vi "main.vi"(0 "Test Pins":T6, 1 "Caller Information":T7, 5 "Test Inputs":T10={"Load Current 1 in A"=0.0, "Load Current 2 in A"=0.0, "Duration of the pulse in Second"=0.5, "Nominal Output Voltage in V"=0.0, "Ref Voltage level for Settling Time Calc"=0.1, "% of Vnom for Settling Time Calc"=10.0, "Settling Time Calc Option"=enum."Voltage Level ", "Advance Setting"={"Prepare"={"Power Test Board.Voltage Level (V)"=6.0, "Power Test Board.Current Limit (A)"=0.1, "Sense Resistance (Ohm)"=1.0, "Fgen.Sample Rate (Sample/s)"=20000000.0}, "Stimulus And Measure"={"Fgen.Offset (V)"=0.0}}, "Save Transient Graph?"=TRUE, "Input Voltage in V"=0.0, "Save Scope Raw Data?"=FALSE, "Delay - t1 in s"=0.25, "Delay - t2 in s"=0.25, "Auto Scale Y-Axis?"=TRUE, "Shunt Resistance (Ohm)"=1.0, "Slew Rate (A/us)"=0.001, "Measure Rising Edge Slew Rate?"=TRUE, "Measure Falling Edge Slew Rate?"=TRUE} {"Advance Setting"."Stimulus And Measure"."Fgen.Offset (V)" min=1.0 format="%#_6p"; "Advance Setting"."Prepare"."Power Test Board.Current Limit (A)" min=1.0 format="%#_6p"; "Advance Setting"."Prepare"."Power Test Board.Voltage Level (V)" min=1.0 format="%#_6p"; "Advance Setting"."Prepare"."Fgen.Sample Rate (Sample/s)" min=1.0 format="%#_6p"; "Advance Setting"."Prepare"."Sense Resistance (Ohm)" min=1.0 format="%#_6p"}, 11 "error in":errorcluster) -> (4 "Test Results":T15 {"Falling Edge - Measured Slew Rate (A/us)" format="%#.5p"; "Rising Edge - Measured Slew Rate (A/us)" format="%#.5p"; "Second Edge - Settling Time in s" format="%#.5p"; "First Edge - Settling Time in s" format="%#.5p"; "Actual Sample Rate in S/s" format="%#.5g"}, 15 "error out":errorcluster)   [LabVIEW 2020, in "LDO Load Transient_AWG.lvlib"]
doc: "<b>Caller</b> Information is input for framework components. Mode should be set to <b>Automation</b> when running from TestStand. Sequence Context should be set to <b>ThisContext</b> when running from TestStand. The values will be updated everytime the setting is applied using \"Edit\" dialog.\n\n<b>Test Pins</b> is names of pins available in the pinmap file. Provide the right pins for the required functionality.\n\n<b>Test Inputs</b> is input required for the measurement to perform.\n\n<b>error in</b> is meant for the sequencing. <b>error in</b> should be <b>no error</b> always.\n\n<b>Test Results</b> contains all the measured data during the measurement and processed results.\n\n<b>error out</b> contains the error occured during measurement.\n\nCheck measurement documentation for more information (<Program Files>\\Soliton Technologies\\MeasurementSuite\\CodeModules\\LDO\\LDO Load Transient.pdf)"
uses:
  LDO Load Transient_AWG.lvlib
  Typedefs/Test Results.ctl
  Typedefs/Test Inputs.ctl
  Typedefs/Settling Time Calc Option.ctl
  Typedefs/Advance Settings.ctl
  Typedefs/Adv Settings Setup Instr.ctl
  Typedefs/Adv Settings Stimulus and Measure.ctl
  <userlib>/_Soliton/Measurement Suite/Reusables/Plugin Common/Typedefs/Caller Events.ctl
  <userlib>/_Soliton/Measurement Suite/Reusables/Plugin Common/Typedefs/Caller Information.ctl
  <userlib>/_Soliton/Measurement Suite/Reusables/Plugin Common/Typedefs/Caller Mode.ctl
  Typedefs/Test Pins.ctl
  Typedefs/Pin Dropdown.ctl
  <userlib>/_Soliton/Measurement Suite/Reusables/Plugin Common/Typedefs/Termination Monitor Info.ctl
  Reusables/UI/Progress Monitor/Progress Monitor Option.ctl
  <vilib>/Utility/miscctls.llb/LVMajorAndMinorColorsTypeDef.ctl
  <instrlib>/niDCPower/nidcpower.llb/niDCPower Source Mode.ctl
  <instrlib>/niDCPower/nidcpower.llb/niDCPower Output Function.ctl
  <instrlib>/niDCPower/nidcpower.llb/niDCPower Wait For Event - Event.ctl
  <instrlib>/niFgen/niFgen.llb/niFgen Trigger Mode.ctl
  <instrlib>/niFgen/niFgen.llb/niFgen Output Mode.ctl
  Typedefs/Transient Configuration.ctl
  <instrlib>/niScope/Controls/niScope scalar measurement.ctl
  <vilib>/Utility/error.llb/DialogType.ctl
  c0d3c9e0-367a-4754-9b2e-773ed4fafa93.vi
  d648f1df-a8d9-4085-9eb0-24252e83c66e.vi
  98c31a9a-65c4-404a-8d29-5fef3c3d30dc.vi
  293d3250-dd4c-4630-9c2a-ad0ba4e4c4de.vi
  e89c743e-5273-4ded-a4f4-1d44fefc8133.vi
  44f97677-0516-4608-8e28-d738a12fef77.vi
  01e50ca5-2bbf-454e-9d2d-d5f5dbc62a55.vi
  49732470-67c5-4264-8b59-91d7a6bf13ef.vi
  29f2f23f-c0b0-483c-8177-98a50cbfcdf1.vi
  a7f9c5ee-455a-46a4-a79d-0a7db08c4ebb.vi
  bb3e62c4-a2c2-4505-9438-f842dd651d6c.vi
  ce2ee1e5-697c-4608-b941-8c9b0f21ffd9.vi
  217e438d-a1ad-49ce-9dcd-d015b5ab8206.vi
  3210b59a-1980-40a2-8b26-190a43568d65.vi
  eadbd7cd-77f9-412a-9e87-0f7f53d679d4.vi
  <userlib>/_Soliton/Measurement Suite/Reusables/InstrumentSessionAPIs/SessionManagerApiPath.vi
  <vilib>/Utility/sysdir.llb/Get System Directory.vi
  <vilib>/Utility/LVLibp/Get Exported File Path.vi
  <userlib>/_Soliton/Measurement Suite/Reusables/Errors/Error 6001.vi
  <instrlib>/niScope/Measurements/niScope Fetch Measurement.vi
  <userlib>/_Soliton/Measurement Suite/Reusables/Plugin Common/Plugin Common.lvlib
  <userlib>/_Soliton/Measurement Suite/Reusables/Queue Driver/Plugin Queue Driver.lvlib
panel:
  out "Progress":i32(slide) scale=-1.0..17.0
  in  "Terminate":bool
  in  "Run":bool caption="Measure"
  in  "Exit":bool
  out "Header":string
  in  "Tab Enum":T1(radio)
  out "Tab Control":T2(tab)
  in  "SystemSetup":T4={"Power test Board"={"PinStatus"=0, "PinName"="", "Info"=TRUE}, "Set Input Voltage"={"PinStatus"=0, "PinName"="", "Info"=TRUE}, "Measure Output Voltage"={"PinStatus"=0, "PinName"="", "Info"=TRUE}, "Measure Load Current"={"PinStatus"=0, "PinName"="", "Info"=TRUE}, "Set Arbitrary Waveform"={"PinStatus"=0, "PinName"="", "Info"=TRUE}}
  in  "Shunt Resistance (Ohm)":dbl=1.0 min=1.0 format="%#_6p"
  out "Shunt Resistance Info":u16(ring) caption="Set 1 Ohm if its Current Probe"
  in  "Slew Rate (A/us)":dbl format="%#_6p"
  out "Sequence Timeout":dbl caption="Sequence Timeout (s)" format="%#.5p"
  in  "Delay - t2 (s)":dbl=0.25 format="%#_6p"
  in  "Delay - t1 (s)":dbl=0.25 format="%#_6p"
  in  "Duration of the pulse (s)":dbl=0.5 format="%#_6p"
  in  "Percentage of Vnom (%)":dbl=10.0 caption="Percentage of nominal voltage (%)" format="%#_6f"
  in  "Voltage to settle above Vnom (V)":dbl=0.1 format="%#_6p"
  in  "Load Current 1 - Iload1 (A)":dbl format="%#_6p"
  in  "Settling Time Calculation":enum32{"Item 0", "Item 1"}(radio)
  in  "Input Voltage (V)":dbl format="%#_6p"
  in  "Load Current 2 - Iload2 (A)":dbl format="%#_6p"
  in  "Nominal Output Voltage (V)":dbl format="%#_6p"
  in  "Advanced Settings":bool
  in  "Measure Falling Edge Slew Rate?":bool=TRUE
  in  "Measure Rising Edge Slew Rate?":bool=TRUE
  out "Falling Edge - Measured Slew Rate (A/us)":dbl format="%#.5p"
  out "Rising Edge - Measured Slew Rate (A/us)":dbl format="%#.5p"
  out "Second Edge - Settling Time (s)":dbl format="%#.5p"
  in  "Auto Scale Y-Axis?":bool=TRUE
  in  "Save Scope Raw Data?":bool=TRUE
  out "Load Transient":cluster{"x-axis":dbl[], "wfm":dbl[]}[](graph)
  in  "Take Transient snapshot?":bool=TRUE
  out "Transient Load Current":waveform(dbl)(graph)
  out "Transient Output Voltage":T5(graph)
  out "First Edge - Settling Time (s)":dbl format="%#.5p"
  out "Rising Edge not found?":bool
  out "Falling Edge not found?":bool
  in  "Caller Events":T9
  in  "DataLogPath":path
  in  "ErrorOccured":errorcluster
  # "Supports NIScopeInstrument"
  # "Supports NIScopeInstrument"
  # "Supports NIDCPowerInstrument"
  # "Supports NIFGenInstrument"
  # "Supports NIDCPowerInstrument"
  # "Load Current"
  # "Minimum value for Delay-t1, Duration of the pulse, Delay-t2 should be larger than [ ( Souredelay+Aperture Time ) x Record Length ]"
  # "Settling Time Calculation"
  # "Settling Time is defined as the time taken for the output voltage to recover\nto the LDO nominal output voltage."
  # "Time taken for output voltage to settle to (Choose one below)"
  # "Load Transient"
  # "Output Voltage"
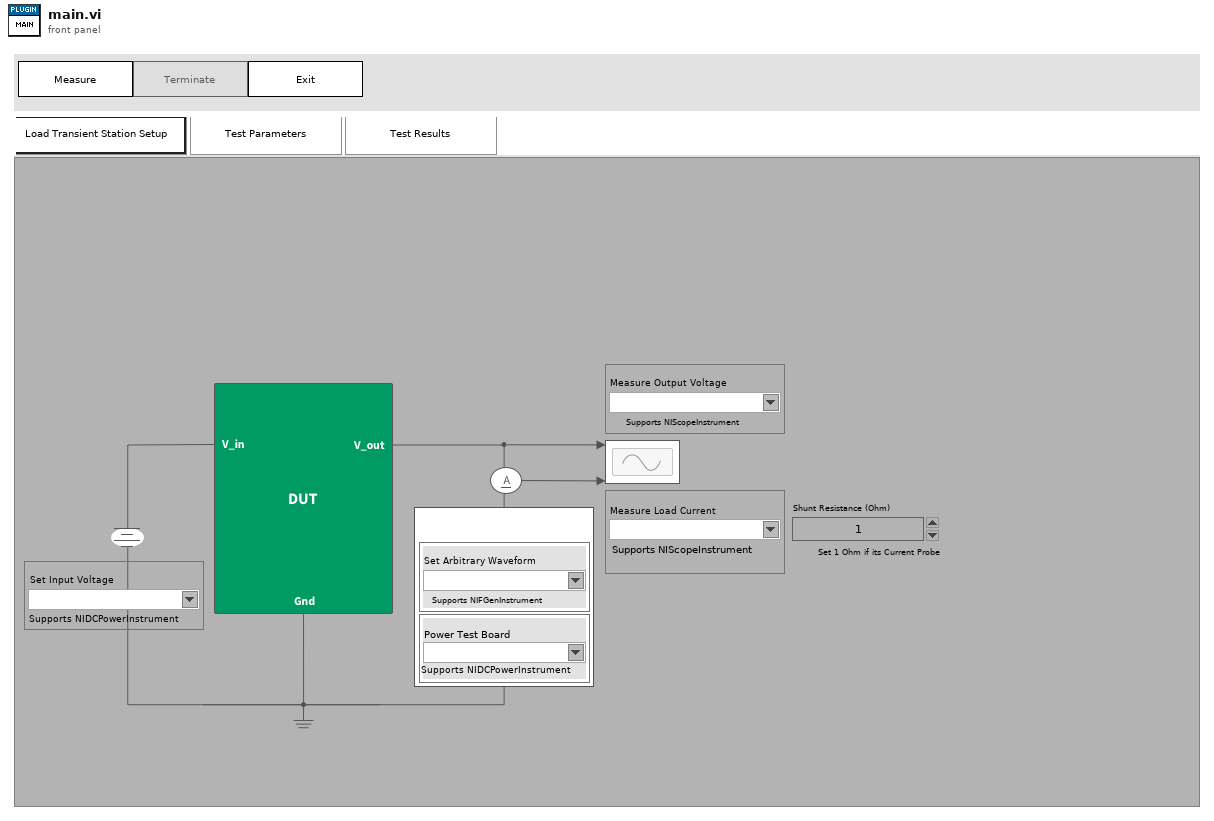
[diagram p1: front panel]
types:
  T1 = enum32{"Station Setup", "Test Parameters", "Test Results"}
  T2 = enum32{"Station Setup", "Test Parameters", "Test Results", "Debug"}
  T3 = typedef "LDO Load Transient_AWG.lvlib/Pin Dropdown.ctl" = cluster{"PinStatus":u16, "PinName":string, "Info":bool}
  T4 = cluster{"Power test Board":T3, "Set Input Voltage":T3, "Measure Output Voltage":T3, "Measure Load Current":T3, "Set Arbitrary Waveform":T3}
  T5 = cluster{"relativeInitialX":dbl, "xIncrement":dbl, "wfm":dbl[]}
  T6 = typedef "LDO Load Transient_AWG.lvlib/Test Pins.ctl" = cluster{"Set Input Voltage":string, "Set Load Current":string, "Set Arbitrary Waveform":string, "Measure Output Voltage":string, "Measure Load Current":string}
  T7 = typedef "Plugin Common.lvlib/Caller Information.ctl" = cluster{"Mode":T8, "Sequence Context":refnum<k7>}
  T8 = typedef "Plugin Common.lvlib/Caller Mode.ctl" = enum16{"Standalone", "Automation", "MeasurementSuite"}
  T9 = typedef "Plugin Common.lvlib/Caller Events.ctl" = cluster{"Caller Event":refnum<user-event>}
  T10 = typedef "LDO Load Transient_AWG.lvlib/Test Inputs.ctl" = cluster{"Load Current 1 in A":dbl, "Load Current 2 in A":dbl, "Duration of the pulse in Second":dbl, "Nominal Output Voltage in V":dbl, "Ref Voltage level for Settling Time Calc":dbl, "% of Vnom for Settling Time Calc":dbl, "Settling Time Calc Option":T11, "Advance Setting":T12, "Save Transient Graph?":bool, "Input Voltage in V":dbl, "Save Scope Raw Data?":bool, "Delay - t1 in s":dbl, "Delay - t2 in s":dbl, "Auto Scale Y-Axis?":bool, "Shunt Resistance (Ohm)":dbl, "Slew Rate (A/us)":dbl, "Measure Rising Edge Slew Rate?":bool, "Measure Falling Edge Slew Rate?":bool}
  T11 = typedef "LDO Load Transient_AWG.lvlib/Settling Time Calc Option.ctl" = enum16{"Voltage Level ", "Percentage of Vnom"}
  T12 = typedef "LDO Load Transient_AWG.lvlib/Advance Settings.ctl" = cluster{"Prepare":T13, "Stimulus And Measure":T14}
  T13 = typedef "LDO Load Transient_AWG.lvlib/Adv Settings Setup Instr.ctl" = cluster{"Power Test Board.Voltage Level (V)":dbl, "Power Test Board.Current Limit (A)":dbl, "Sense Resistance (Ohm)":dbl, "Fgen.Sample Rate (Sample/s)":dbl}
  T14 = typedef "LDO Load Transient_AWG.lvlib/Adv Settings Stimulus and Measure.ctl" = cluster{"Fgen.Offset (V)":dbl}
  T15 = typedef "LDO Load Transient_AWG.lvlib/Test Results.ctl" = cluster{"Measured Output Voltage":cluster{"x-axis":dbl[], "wfm":dbl[]}, "Measured Load Current":cluster{"x-axis":dbl[], "wfm":dbl[]}, "Actual Sample Rate in S/s":dbl, "First Edge - Settling Time in s":dbl, "Second Edge - Settling Time in s":dbl, "Rising Edge - Measured Slew Rate (A/us)":dbl, "Falling Edge - Measured Slew Rate (A/us)":dbl}
  T16 = typedef "Plugin Common.lvlib/Termination Monitor Info.ctl" = cluster{"Caller Information":T7, "Execution":refnum<k7>, "Termination Monitor":refnum<k7>, "Type":string, "Plugin Name":string}
  T17 = cluster{"Termination Monitor Info":T16, "Test Inputs":T10, "Test Results":T15, "Test Results[][]":string[][], "Test Pins":T6, "Logger Folder Path":path, "Valid Logger Path?":bool, "Logger File Path":path, "Min delay for Reference Position":u32, "Output Voltage Coupling":i32, "UI Ctls":refnum<vi>[], "Insufficient memory?":bool, "Scope Channels":string, "Scope Acquired time(s)":dbl, "Rising Edge not found?":bool, "Falling Edge not found?":bool}
  T18 = typedef "Progress Monitor Option.ctl" = enum16{"State Array Init", "Get State Index"}
  T19 = enum8{"Enabled", "Disabled", "Disabled and Grayed Out"}
  T20 = typedef "LDO Load Transient_AWG.lvlib/Transient Configuration.ctl" = cluster{"Delay - t1 (s)":dbl, "Duration of the pulse (s)":dbl, "Delay - t2 (s)":dbl, "Load Current 1 - Iload1 (A)":dbl, "Load Current 2 - Iload2 (A)":dbl, "Slew rate A/us":dbl, "Sense Resistance (Ohm)":dbl}
  T21 = typedef "LVMajorAndMinorColorsTypeDef.ctl" = cluster{"Major Color":u32, "Minor Color":u32}
  T22 = typedef "niDCPower Wait For Event - Event.ctl" = i32
  T23 = typedef "niDCPower Output Function.ctl" = i32
  T24 = typedef "niDCPower Source Mode.ctl" = i32
  T25 = typedef "niFgen Output Mode.ctl" = u32
  T26 = typedef "niFgen Trigger Mode.ctl" = i32
  T27 = typedef "niScope scalar measurement.ctl" = i32
  T28 = typedef "DialogType.ctl" = u16
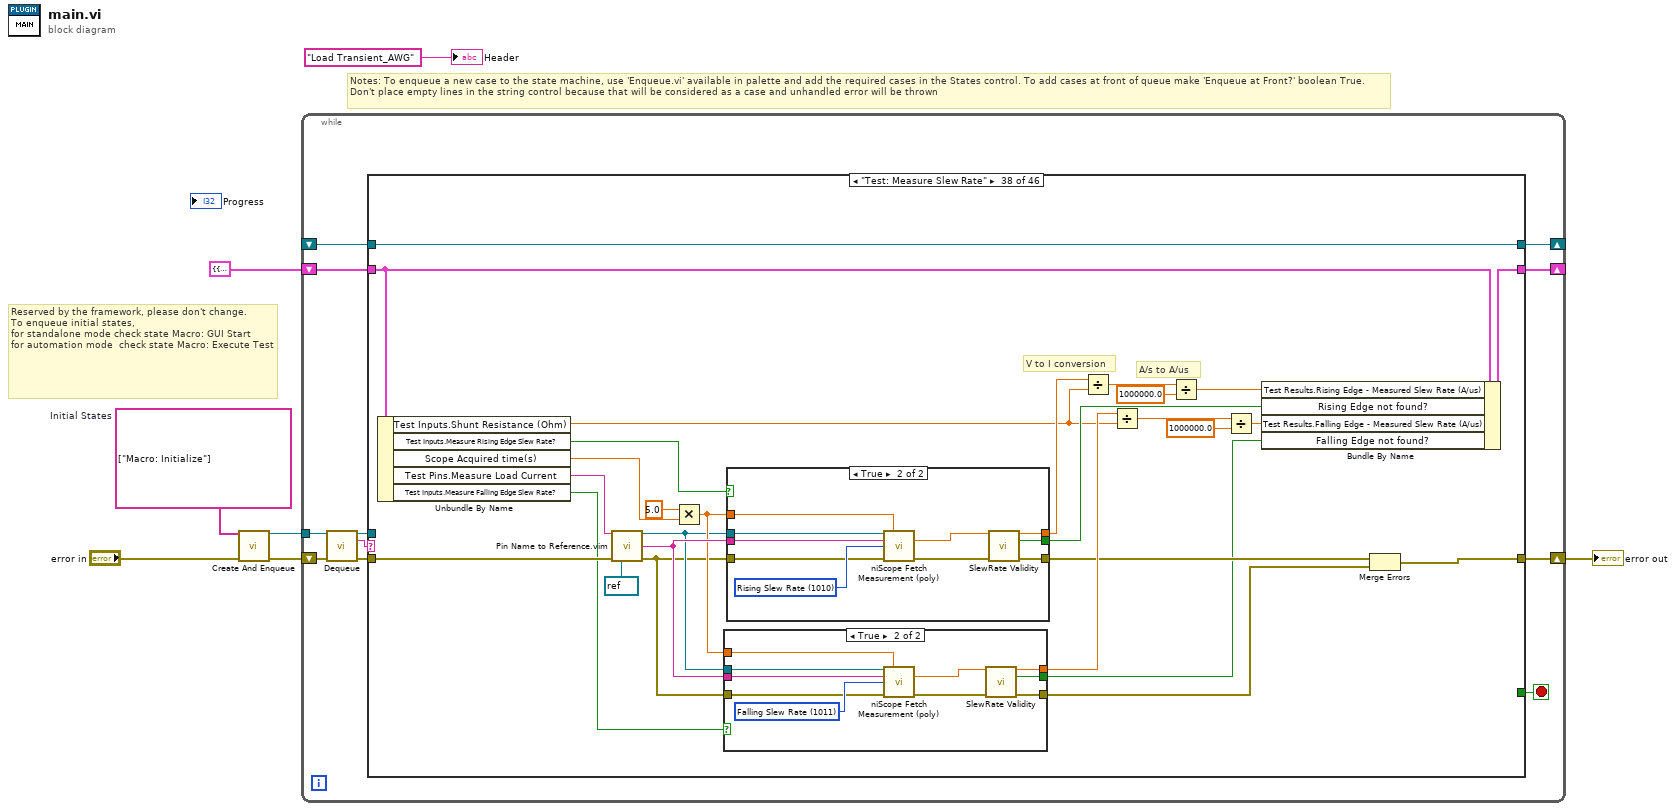
[diagram p0: block diagram]
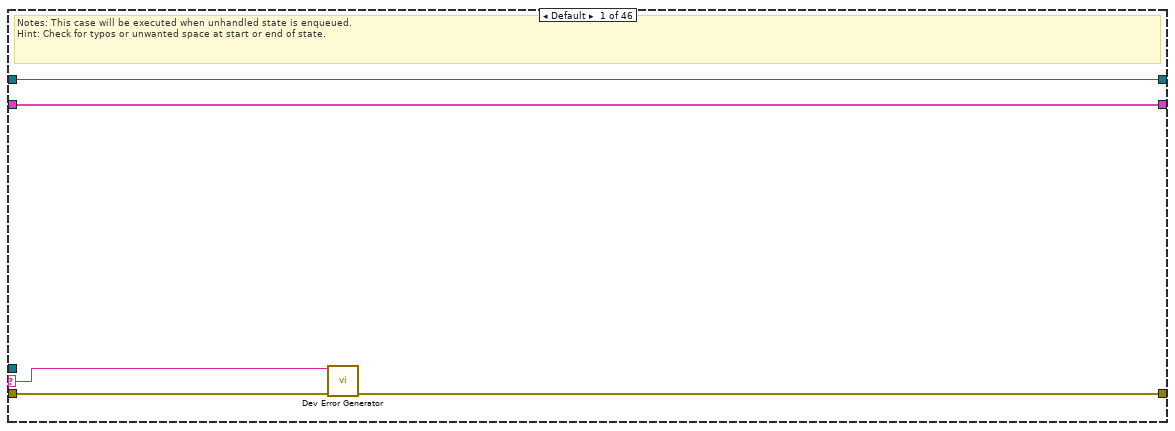
[diagram p2: hidden frame]
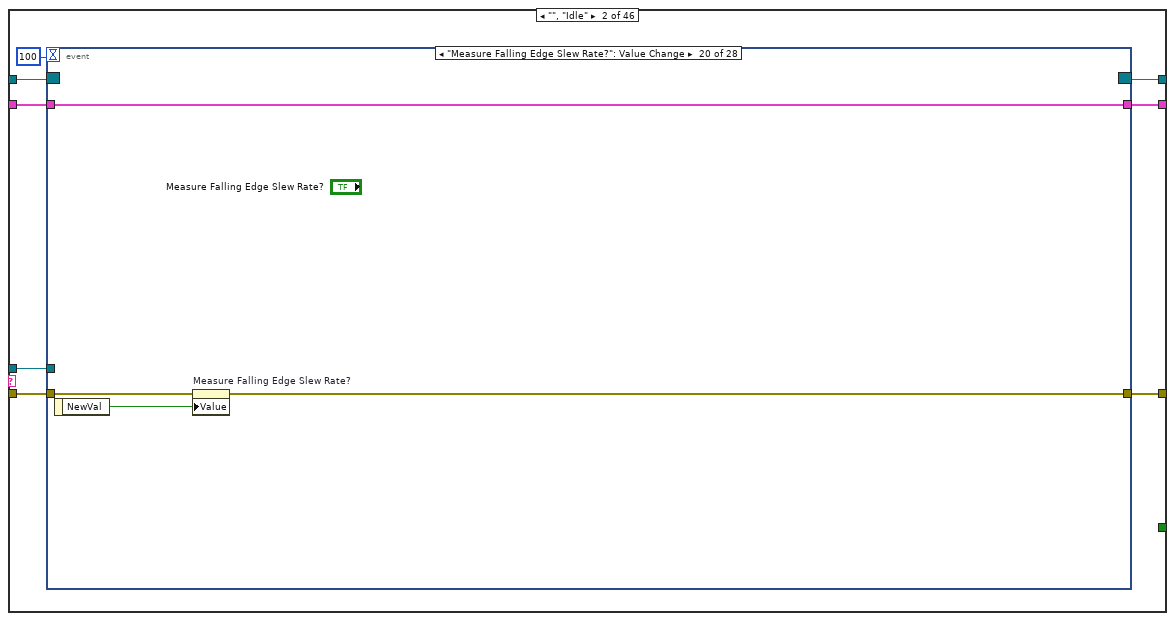
[diagram p3: hidden frame]
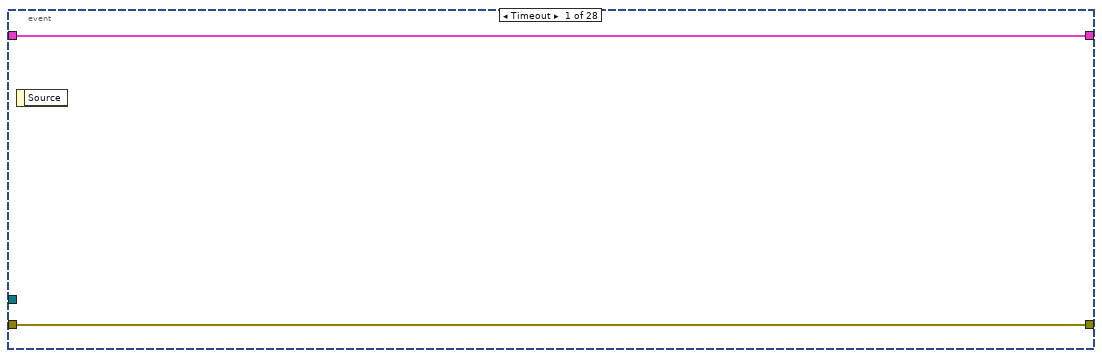
[diagram p4: hidden frame]
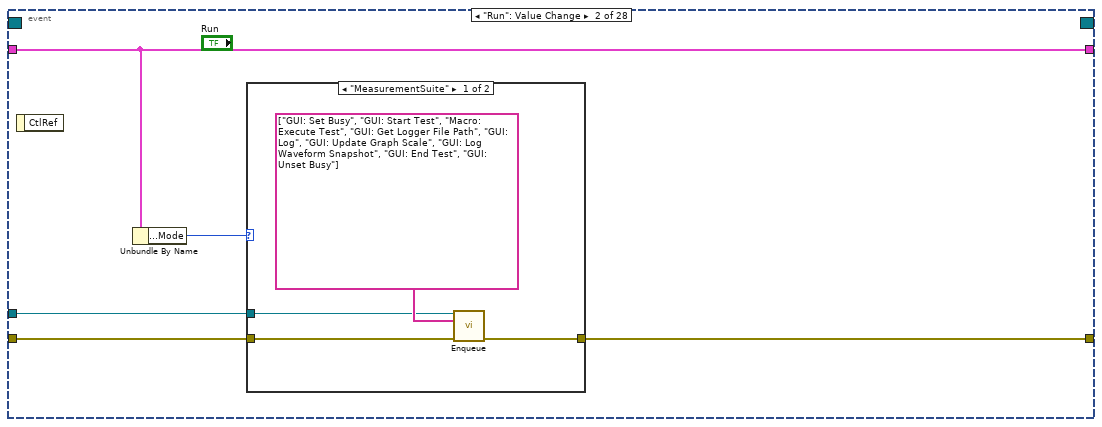
[diagram p5: hidden frame]
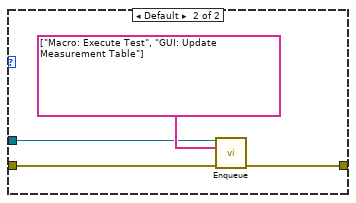
[diagram p6: hidden frame]
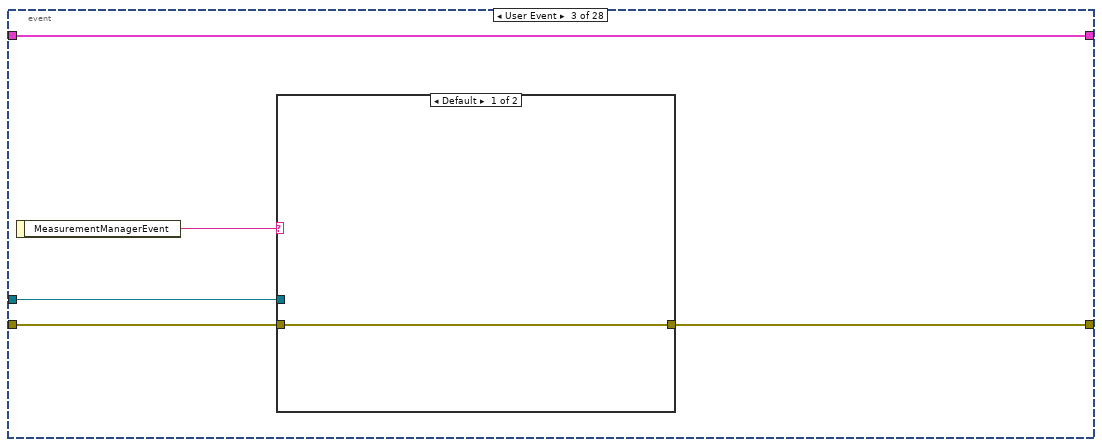
[diagram p7: hidden frame]
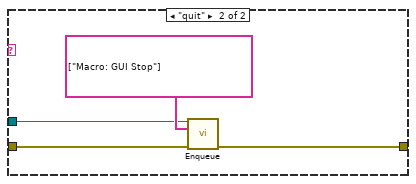
[diagram p8: hidden frame]
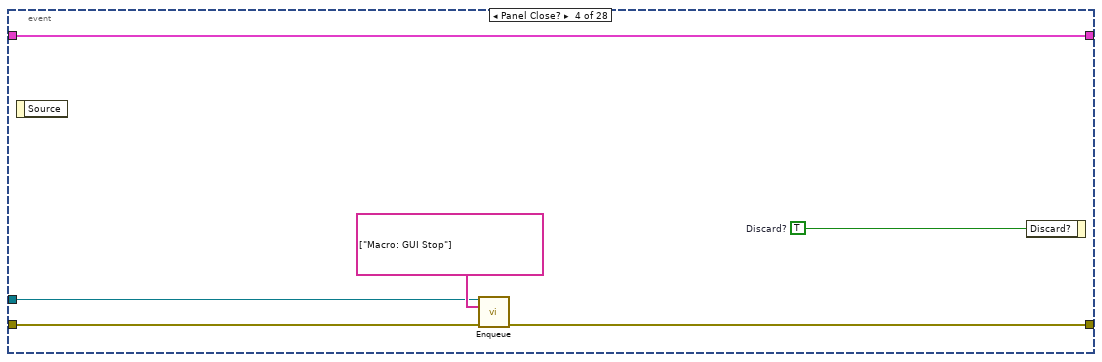
[diagram p9: hidden frame]
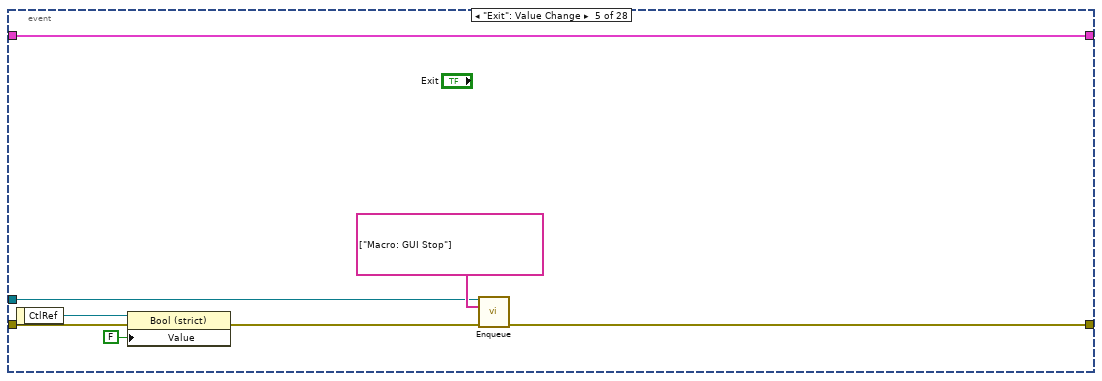
[diagram p10: hidden frame]
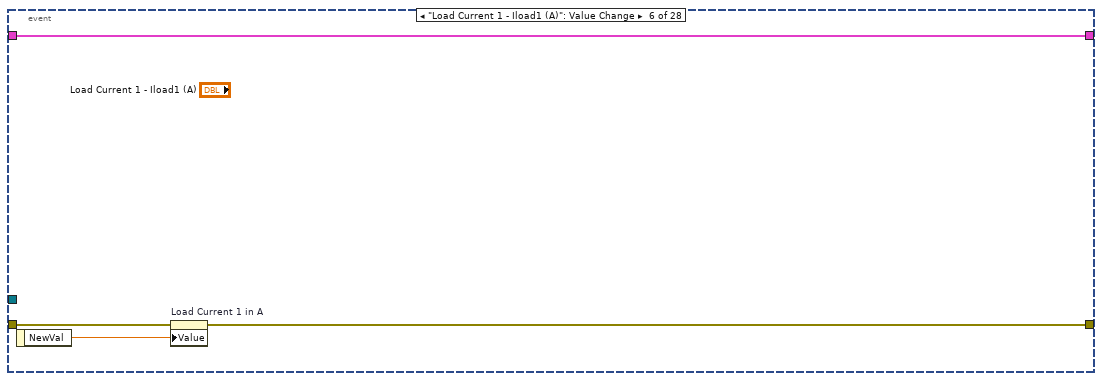
[diagram p11: hidden frame]
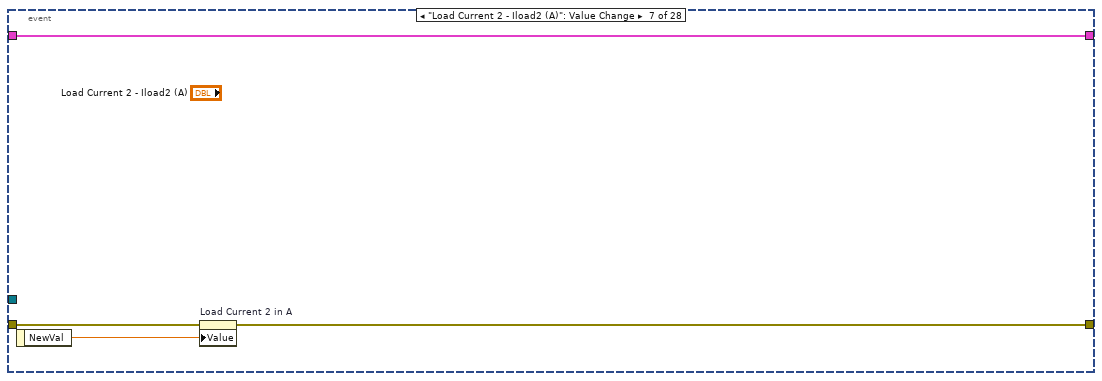
[diagram p12: hidden frame]
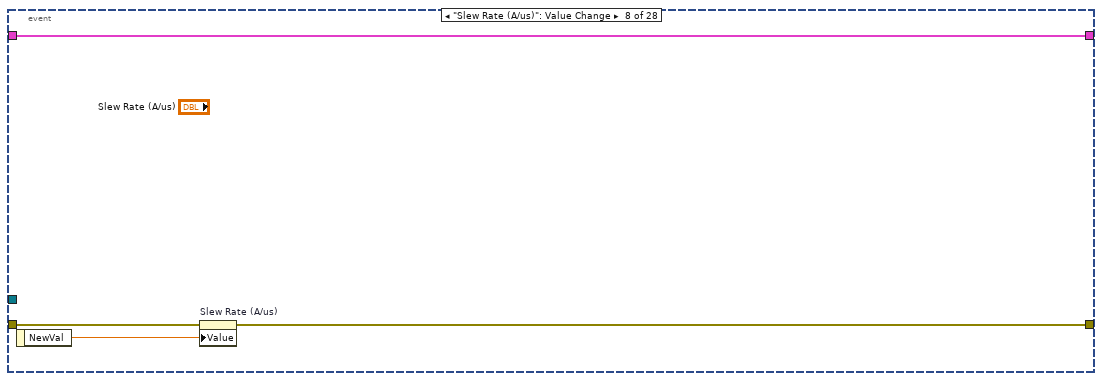
[diagram p13: hidden frame]
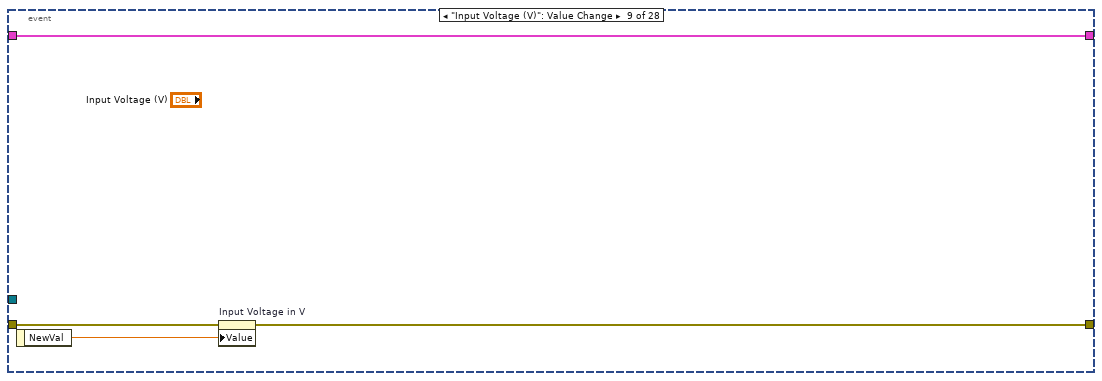
[diagram p14: hidden frame]
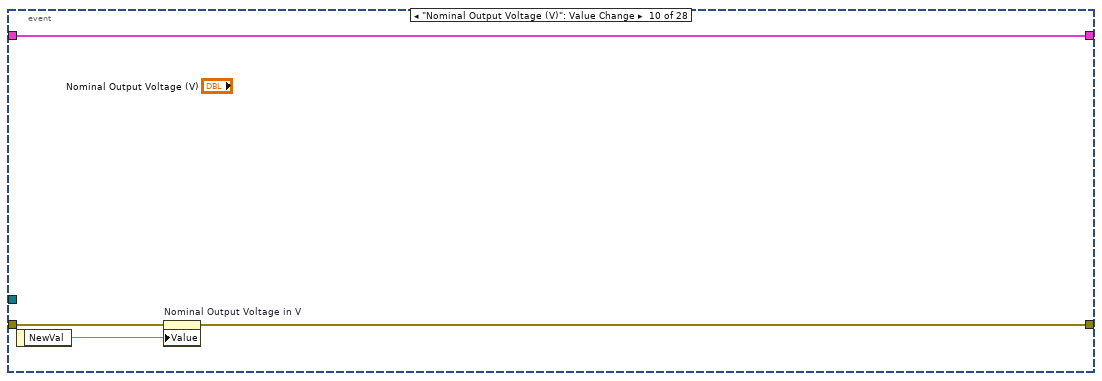
[diagram p15: hidden frame]
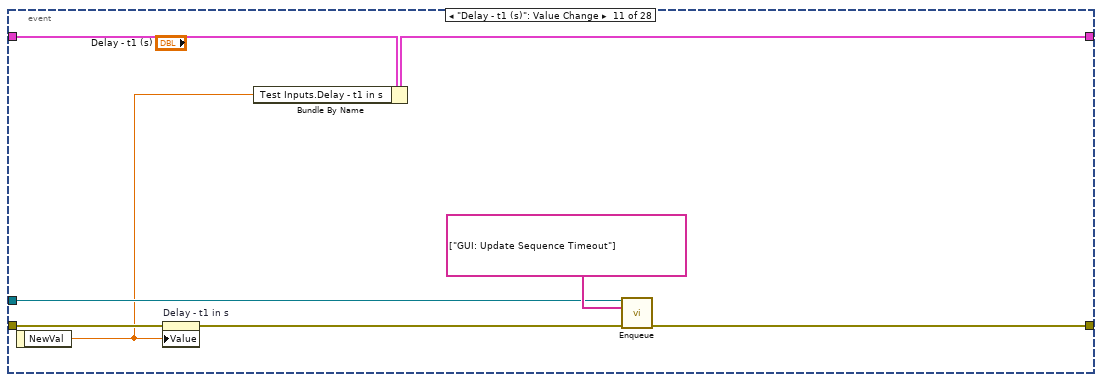
[diagram p16: hidden frame]
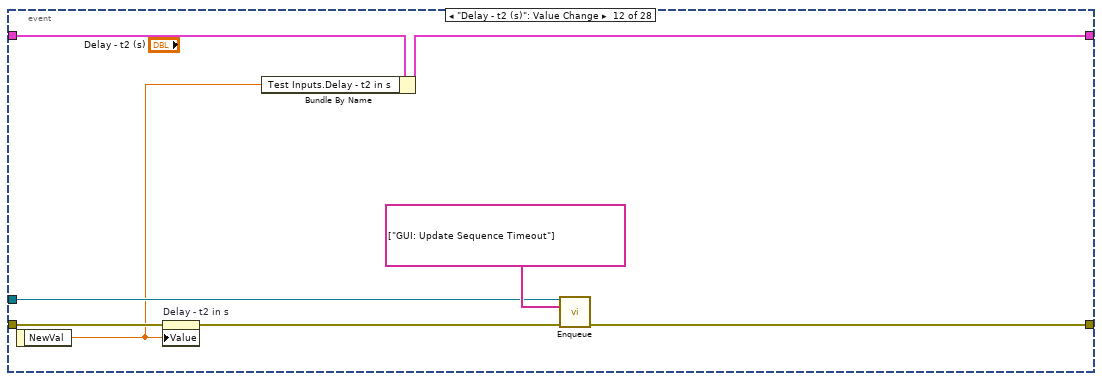
[diagram p17: hidden frame]
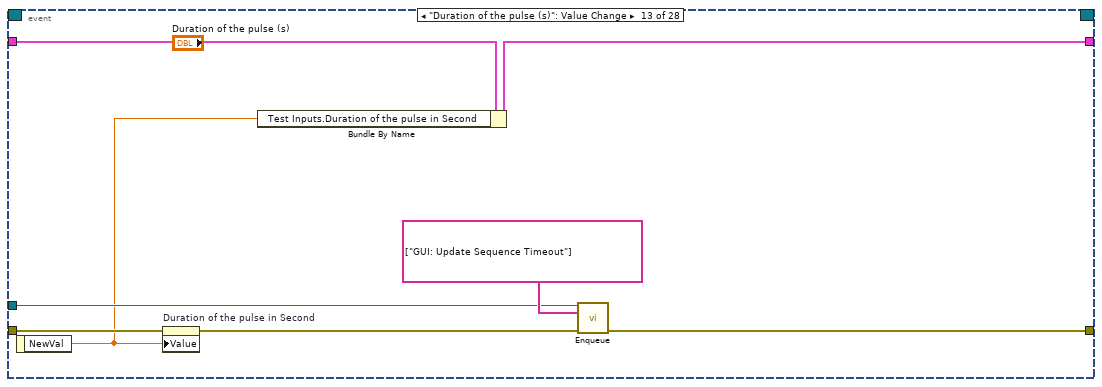
[diagram p18: hidden frame]
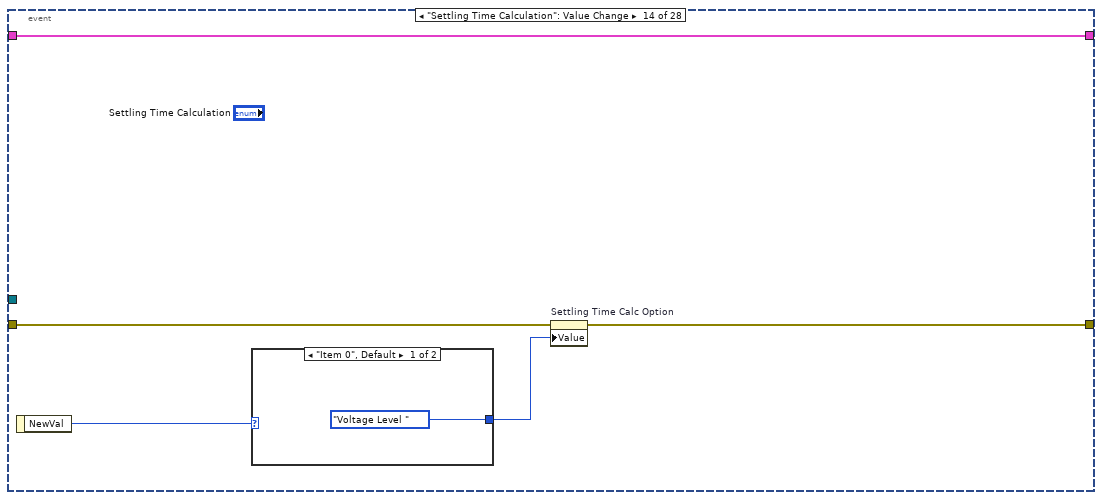
[diagram p19: hidden frame]
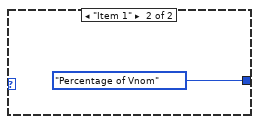
[diagram p20: hidden frame]
diagram:
  w7 = string[] ["Macro: Initialize"]  # Initial States
  # "Notes: To enqueue a new case to the state machine, use 'Enqueue.vi' available in palette and add the required cases in the States control. To add cases at front of queue make 'Enqueue at Front?' boolean True. Don't place empty lines in the string control because that will be considered as a case and unhandled error will be thrown"
  # "Reserved by the framework, please don't change. \nTo enqueue initial states,\nfor standalone mode check state Macro: GUI Start\nfor automation mode  check state Macro: Execute Test"
  n1 = call <userlib>:"Create And Enqueue.vi"("Initial States"=w7, "error in (no error)"="error in") -> ("Queue out"=w5:refnum<queue>, "error out"=w3:errorcluster)  [unwired: 12 in]
  n2 = while {
    shift-right: [w18] -> w4
    shift-left: w3 -> [w16]
    shift-right: [w14] -> _
    shift-left: T17 {"Termination Monitor Info"={"Caller Information"={"Mode"=enum."Standalone", "Sequence Context"=refnum}, "Execution"=refnum, "Termination Monitor"=refnum, "Type"="", "Plugin Name"=""}, "Test Inputs"={"Load Current 1 in A"=0.0, "Load Current 2 in A"=0.0, "Duration of the pulse in Second"=0.0, "Nominal Output Voltage in V"=0.0, "Ref Voltage level for Settling Time Calc"=0.0, "% of Vnom for Settling Time Calc"=0.0, "Settling Time Calc Option"=enum."Voltage Level ", "Advance Setting"={"Prepare"={"Power Test Board.Voltage Level (V)"=0.0, "Power Test Board.Current Limit (A)"=0.0, "Sense Resistance (Ohm)"=1.0, "Fgen.Sample Rate (Sample/s)"=1.0}, "Stimulus And Measure"={"Fgen.Offset (V)"=0.0}}, "Save Transient Graph?"=FALSE, "Input Voltage in V"=0.0, "Save Scope Raw Data?"=FALSE, "Delay - t1 in s"=0.0, "Delay - t2 in s"=0.0, "Auto Scale Y-Axis?"=FALSE, "Shunt Resistance (Ohm)"=0.0, "Slew Rate (A/us)"=0.0, "Measure Rising Edge Slew Rate?"=TRUE, "Measure Falling Edge Slew Rate?"=TRUE}, "Test Results"={"Measured Output Voltage"={"x-axis"=[], "wfm"=[]}, "Measured Load Current"={"x-axis"=[], "wfm"=[]}, "Actual Sample Rate in S/s"=0.0, "First Edge - Settling Time in s"=0.0, "Second Edge - Settling Time in s"=0.0, "Rising Edge - Measured Slew Rate (A/us)"=0.0, "Falling Edge - Measured Slew Rate (A/us)"=0.0}, "Test Results[][]"=[], "Test Pins"={"Set Input Voltage"="", "Set Load Current"="", "Set Arbitrary Waveform"="", "Measure Output Voltage"="", "Measure Load Current"=""}, "Logger Folder Path"=path "", "Valid Logger Path?"=FALSE, "Logger File Path"=path "", "Min delay for Reference Position"=0, "Output Voltage Coupling"=0, "UI Ctls"=[], "Insufficient memory?"=FALSE, "Scope Channels"="", "Scope Acquired time(s)"=0.0, "Rising Edge not found?"=FALSE, "Falling Edge not found?"=FALSE} -> [w13]
    tunnel: w5 -> [w12]
    shift-right: [w9] -> _
    shift-left: _ -> [w10]
    stop <- w17 stop-if-true
    n3 = call <userlib>:"Dequeue.vi"("Queue in"=w12, "error in (no error)"=w16) -> ("Queue out"=w11:refnum<queue>, "Dequeued State"=w8:string, "error out"=w15:errorcluster)  [unwired: 11 in]
    n4 = case shown="\"Test: Measure Slew Rate\"" w8 {
      selector: w8 -> [w21 _ _ _ _ _ _ _ _ _ _ _ w351 w367 _ _ _ _ _ _ _ _ _ _ _ w529 w549 w582 w613 _ _ w673 w680 w728 w767 w790 w806 _ w889 w906 w924 w940 w949 _ _ _]
      tunnel: w15 -> [w20 w28 w255 w264 w279 w285 w292 w297 w332 w343 w347 w350 w352 w369 w384 w396 w425 w438 w459 w491 w500 w511 w516 w523 w528 w530 w550 w583 w614 w634 w657 w674 w681 w729 w768 w791 w807 w846 w890 w907 w925 w941 w950 w957 w964 w982]
      tunnel: [w22 w29 w255 w267 w270 w286 w293 w297 w298 w341 w345 w350 w356 w372 w385 w395 w426 w436 w460 w492 w499 w511 w517 w524 w528 w536 w548 w562 w617 w620 w658 w672 w688 w714 w764 w792 w808 w830 w883 w910 w919 w942 w951 w957 w962 w976] -> w18
      tunnel: [_ _ _ _ _ _ _ _ _ _ _ _ _ _ _ _ _ _ _ _ _ _ _ _ _ _ _ _ _ _ _ _ _ _ _ _ _ _ _ _ _ _ _ _ w959 TRUE] -> w17
      tunnel: [w23 w31 w254 w257 w280 w287 w294 w296 w323 w342 w346 w349 w355 w371 w391 w394 w427 w452 w458 w498 w508 w510 w515 w522 w527 w535 w553 w585 w612 w637 w660 w677 w685 w731 w771 w795 w811 w839 w895 w912 w929 w947 w954 w956 w961 w983] -> w14
      tunnel: w13 -> [w23 w30 w254 w268 w280 w287 w294 w296 w337 w342 w346 w349 w355 w371 w391 w393 w427 w452 w458 w498 w508 w510 w514 w521 w527 w545 w553 w585 w611 w637 w659 w677 w684 w731 w770 w794 w810 w838 w895 w912 w929 w947 w954 w956 w961 w983]
      tunnel: w11 -> [_ w24 _ w266 w278 w283 w290 _ _ _ _ _ _ _ _ _ _ _ _ _ _ _ _ _ _ _ _ _ _ _ _ _ _ _ _ _ _ _ _ _ _ _ _ _ w958 w981]
      tunnel: w10 -> [w19 w26 w253 w265 w277 w282 w289 w295 w336 _ w344 w348 w362 w378 w392 w401 w428 w453 w465 w497 w507 w509 w518 w525 w526 w543 w554 w586 w619 w638 w661 w678 w689 w732 w772 w801 w820 w848 w896 w917 w932 w948 w953 w955 w963 w980]
      tunnel: [w19 w25 w253 w265 w277 w282 w289 w295 w336 w340 w344 w348 w362 w378 w392 w401 w428 w453 w465 w497 w507 w509 w518 w525 w526 w543 w554 w586 w619 w638 w661 w678 w689 w732 w772 w801 w820 w848 w896 w917 w932 w948 w953 w955 w963 w980] -> w9
      frame Default {
        # "Notes: This case will be executed when unhandled state is enqueued. \nHint: Check for typos or unwanted space at start or end of state."
        n5 = call <userlib>:"Dev Error Generator.vi"("State"=w21, "error in (no error)"=w20) -> ("error out"=w22:errorcluster)  [unwired: 13 in]
      }
      frame "", "Idle" {
        n6 = event shown="[19] \"Measure Falling Edge Slew Rate?\": Value Change" {
          selector: w26 -> [_ _ _ _ _ _ _ _ _ _ _ _ _ _ _ _ _ _ _ _ _ _ _ _ _ _ _ _]
          dyn-events: [_ _ _ _ _ _ _ _ _ _ _ _ _ _ _ _ _ _ _ _ _ _ _ _ _ _ _ _] -> w25
          timeout: 100 -> [_ _ _ _ _ _ _ _ _ _ _ _ _ _ _ _ _ _ _ _ _ _ _ _ _ _ _ _]
          tunnel: [w33 w35 w51 w62 w70 w74 w78 w82 w86 w90 w93 w101 w109 w119 w127 w138 w149 w153 w157 w161 w165 w171 w179 w191 w236 w241 w246 w252] -> w31
          tunnel: w30 -> [w33 w35 w51 w62 w70 w74 w78 w82 w86 w90 w92 w100 w108 w119 w127 w138 w149 w153 w157 w161 w165 w173 w178 w190 w235 w241 w245 w252]
          tunnel: [w32 w38 w49 w59 w68 w73 w77 w81 w84 w89 w95 w103 w111 w116 w125 w135 w147 w151 w155 w159 w163 w167 w180 w184 w218 w240 w243 w250] -> w29
          tunnel: w28 -> [w32 w37 w50 w58 w67 w72 w76 w80 w85 w88 w98 w106 w114 w117 w126 w134 w148 w152 w156 w160 w164 w172 w180 w193 w217 w240 w248 w251]
          tunnel: w24 -> [_ w36 w47 w57 w66 _ _ _ _ _ w94 w102 w110 _ _ _ _ _ _ _ _ _ _ _ _ _ _ _]
          event Timeout {
            n7 = event-data() -> ()  [unwired: 1 in, 1 out]
          }
          event "Run": Value Change {
            n8 = event-data() -> ()  [unwired: 1 in, 1 out]
            n9 = Unbundle By Name(w35) -> ("Termination Monitor Info.Caller Information.Mode"=w34:T8)
            n10 = case shown="\"MeasurementSuite\"" w34 {
              tunnel: [w41 w45] -> w38
              tunnel: w37 -> [w40 w44]
              tunnel: w36 -> [w39 w43]
              frame "MeasurementSuite" {
                n11 = call <userlib>:"Enqueue.vi"("Queue in"=w39, "States"=string[] ["GUI: Set Busy", "GUI: Start Test", "Macro: Execute Test", "GUI: Get Logger File Path", "GUI: Log", "GUI: Update Graph Scale", "GUI: Log Waveform Snapshot", "GUI: End Test", "GUI: Unset Busy"], "error in (no error)"=w40) -> ("error out"=w41:errorcluster)  [unwired: 11 in, 1 out]
              }
              frame Default {
                n12 = call <userlib>:"Enqueue.vi"("Queue in"=w43, "States"=string[] ["Macro: Execute Test", "GUI: Update Measurement Table"], "error in (no error)"=w44) -> ("error out"=w45:errorcluster)  [unwired: 11 in, 1 out]
              }
            }
          }
          event User Event {
            n13 = event-data() -> ("MeasurementManagerEvent"=w48:string)  [unwired: 1 in]
            n14 = case shown="Default" w48 {
              tunnel: [w52 w53] -> w49
              tunnel: w50 -> [w52 w55]
              tunnel: w47 -> [_ w54]
              frame Default {
              }
              frame "quit" {
                n15 = call <userlib>:"Enqueue.vi"("Queue in"=w54, "States"=string[] ["Macro: GUI Stop"], "error in (no error)"=w55) -> ("error out"=w53:errorcluster)  [unwired: 11 in, 1 out]
              }
            }
          }
          event Panel Close? {
            w61 = TRUE  # Discard?
            n16 = event-data() -> ()  [unwired: 1 in, 1 out]
            n17 = call <userlib>:"Enqueue.vi"("Queue in"=w57, "States"=string[] ["Macro: GUI Stop"], "error in (no error)"=w58) -> ("error out"=w59:errorcluster)  [unwired: 11 in, 1 out]
            n18 = event-data("Discard?"=w61) -> ()  [unwired: 1 in, 1 out]
          }
          event "Exit": Value Change {
            n19 = event-data() -> ("CtlRef"=w64:refnum<vi>)  [unwired: 1 in]
            n20 = property class="Bool (strict)"(reference=w64, error in=w67, "Value"=FALSE) -> (error out=w65:errorcluster)  [unwired: 1 out]
            n21 = call <userlib>:"Enqueue.vi"("Queue in"=w66, "States"=string[] ["Macro: GUI Stop"], "error in (no error)"=w65) -> ("error out"=w68:errorcluster)  [unwired: 11 in, 1 out]
          }
          event "Load Current 1 - Iload1 (A)": Value Change {
            n22 = event-data() -> ("NewVal"=w71:dbl)  [unwired: 1 in]
            n23 = property on="Load Current 1 in A" class="DigNum (strict)"(error in=w72, "Value"=w71) -> (error out=w73:errorcluster)  [unwired: 1 in, 1 out]
          }
          event "Load Current 2 - Iload2 (A)": Value Change {
            n24 = event-data() -> ("NewVal"=w75:dbl)  [unwired: 1 in]
            n25 = property on="Load Current 2 in A" class="DigNum (strict)"(error in=w76, "Value"=w75) -> (error out=w77:errorcluster)  [unwired: 1 in, 1 out]
          }
          event "Slew Rate (A/us)": Value Change {
            n26 = event-data() -> ("NewVal"=w79:dbl)  [unwired: 1 in]
            n27 = property on="Slew Rate (A/us)" class="DigNum (strict)"(error in=w80, "Value"=w79) -> (error out=w81:errorcluster)  [unwired: 1 in, 1 out]
          }
          event "Input Voltage (V)": Value Change {
            n28 = event-data() -> ("NewVal"=w83:dbl)  [unwired: 1 in]
            n29 = property on="Input Voltage in V" class="DigNum (strict)"(error in=w85, "Value"=w83) -> (error out=w84:errorcluster)  [unwired: 1 in, 1 out]
          }
          event "Nominal Output Voltage (V)": Value Change {
            n30 = event-data() -> ("NewVal"=w87:dbl)  [unwired: 1 in]
            n31 = property on="Nominal Output Voltage in V" class="DigNum (strict)"(error in=w88, "Value"=w87) -> (error out=w89:errorcluster)  [unwired: 1 in, 1 out]
          }
          event "Delay - t1 (s)": Value Change {
            n32 = event-data() -> ("NewVal"=w91:dbl)  [unwired: 1 in]
            n33 = property on="Delay - t1 in s" class="DigNum (strict)"(error in=w98, "Value"=w91) -> (error out=w96:errorcluster)  [unwired: 1 in, 1 out]
            n34 = Bundle By Name(cluster=w92, "Test Inputs.Delay - t1 in s"=w91) -> (w93:T17)
            n35 = call <userlib>:"Enqueue.vi"("Queue in"=w94, "States"=string[] ["GUI: Update Sequence Timeout"], "error in (no error)"=w96) -> ("error out"=w95:errorcluster)  [unwired: 11 in, 1 out]
          }
          event "Delay - t2 (s)": Value Change {
            n36 = event-data() -> ("NewVal"=w99:dbl)  [unwired: 1 in]
            n37 = property on="Delay - t2 in s" class="DigNum (strict)"(error in=w106, "Value"=w99) -> (error out=w104:errorcluster)  [unwired: 1 in, 1 out]
            n38 = Bundle By Name(cluster=w100, "Test Inputs.Delay - t2 in s"=w99) -> (w101:T17)
            n39 = call <userlib>:"Enqueue.vi"("Queue in"=w102, "States"=string[] ["GUI: Update Sequence Timeout"], "error in (no error)"=w104) -> ("error out"=w103:errorcluster)  [unwired: 11 in, 1 out]
          }
          event "Duration of the pulse (s)": Value Change {
            n40 = event-data() -> ("NewVal"=w107:dbl)  [unwired: 1 in]
            n41 = property on="Duration of the pulse in Second" class="DigNum (strict)"(error in=w114, "Value"=w107) -> (error out=w112:errorcluster)  [unwired: 1 in, 1 out]
            n42 = Bundle By Name(cluster=w108, "Test Inputs.Duration of the pulse in Second"=w107) -> (w109:T17)
            n43 = call <userlib>:"Enqueue.vi"("Queue in"=w110, "States"=string[] ["GUI: Update Sequence Timeout"], "error in (no error)"=w112) -> ("error out"=w111:errorcluster)  [unwired: 11 in, 1 out]
          }
          event "Settling Time Calculation": Value Change {
            n44 = event-data() -> ("NewVal"=w118:enum32{"Item 0", "Item 1"})  [unwired: 1 in]
            n45 = case shown="\"Item 0\", Default" w118 {
              tunnel: [Settling_Time_Calc_Option."Voltage Level " ("Value") Settling_Time_Calc_Option."Percentage of Vnom" ("Value")] -> w115
              frame "Item 0", Default {
              }
              frame "Item 1" {
              }
            }
            n46 = property on="Settling Time Calc Option" class="Enum (strict)"(error in=w117, "Value"=w115) -> (error out=w116:errorcluster)  [unwired: 1 in, 1 out]
          }
          event "Voltage to settle above Vnom (V)": Value Change {
            n47 = event-data() -> ("NewVal"=w122:dbl)  [unwired: 1 in]
            n48 = local read "Test Inputs"() -> (w124:T10)
            n49 = Unbundle By Name(w124) -> ("Settling Time Calc Option"=w123:T11)
            n50 = case shown="\"Voltage Level \"" w123 {
              tunnel: w126 -> [w130 w131]
              tunnel: [w129 w131] -> w125
              tunnel: w122 -> [w128 _]
              frame "Voltage Level " {
                n51 = property on="Ref Voltage level for Settling Time Calc" class="DigNum (strict)"(error in=w130, "Value"=w128) -> (error out=w129:errorcluster)  [unwired: 1 in, 1 out]
              }
              frame "Percentage of Vnom", Default {
              }
            }
          }
          event "Percentage of Vnom (%)": Value Change {
            n52 = event-data() -> ("NewVal"=w133:dbl)  [unwired: 1 in]
            n53 = local read "Test Inputs"() -> (w136:T10)
            n54 = Unbundle By Name(w136) -> ("Settling Time Calc Option"=w137:T11, "Nominal Output Voltage in V"=w132:dbl)
            n55 = case shown="\"Percentage of Vnom\"" w137 {
              tunnel: w134 -> [w139 w145]
              tunnel: [w139 w141] -> w135
              tunnel: w133 -> [_ w140]
              tunnel: w132 -> [_ w142]
              frame "Voltage Level ", Default {
              }
              frame "Percentage of Vnom" {
                n56 = formula code="y = (x/100)*v;"("v"=w142, "x"=w140) -> ("y"=w143:dbl)
                n57 = property on="Ref Voltage level for Settling Time Calc" class="DigNum (strict)"(error in=w145, "Value"=w143) -> (error out=w144:errorcluster)  [unwired: 1 in, 1 out]
                n58 = property on="% of Vnom for Settling Time Calc" class="DigNum (strict)"(error in=w144, "Value"=w140) -> (error out=w141:errorcluster)  [unwired: 1 in, 1 out]
              }
            }
          }
          event "Take Transient snapshot?": Value Change {
            n59 = event-data() -> ("NewVal"=w146:bool)  [unwired: 1 in]
            n60 = property on="Save Transient Graph?" class="Bool (strict)"(error in=w148, "Value"=w146) -> (error out=w147:errorcluster)  [unwired: 1 in, 1 out]
          }
          event "Save Scope Raw Data?": Value Change {
            n61 = event-data() -> ("NewVal"=w150:bool)  [unwired: 1 in]
            n62 = property on="Save Scope Raw Data?" class="Bool (strict)"(error in=w152, "Value"=w150) -> (error out=w151:errorcluster)  [unwired: 1 in, 1 out]
          }
          event "Measure Rising Edge Slew Rate?": Value Change {
            n63 = event-data() -> ("NewVal"=w154:bool)  [unwired: 1 in]
            n64 = property on="Measure Rising Edge Slew Rate?" class="Bool (strict)"(error in=w156, "Value"=w154) -> (error out=w155:errorcluster)  [unwired: 1 in, 1 out]
          }
          event "Measure Falling Edge Slew Rate?": Value Change {
            n65 = event-data() -> ("NewVal"=w158:bool)  [unwired: 1 in]
            n66 = property on="Measure Falling Edge Slew Rate?" class="Bool (strict)"(error in=w160, "Value"=w158) -> (error out=w159:errorcluster)  [unwired: 1 in, 1 out]
          }
          event "Auto Scale Y-Axis?": Value Change {
            n67 = event-data() -> ("NewVal"=w162:bool)  [unwired: 1 in]
            n68 = property on="Auto Scale Y-Axis?" class="Bool (strict)"(error in=w164, "Value"=w162) -> (error out=w163:errorcluster)  [unwired: 1 in, 1 out]
          }
          event "SystemSetup": Value Change {
            n69 = event-data() -> ("NewVal"=w168:T4)  [unwired: 1 in]
            n70 = Unbundle By Name(w168) -> ("Set Input Voltage.PinName"=w176:string, "Power test Board.PinName"=w175:string, "Measure Output Voltage.PinName"=w174:string, "Measure Load Current.PinName"=w169:string, "Set Arbitrary Waveform.PinName"=w166:string)
            n71 = Bundle By Name(cluster=w173, "Test Pins.Set Input Voltage"=w176, "Test Pins.Set Load Current"=w175, "Test Pins.Measure Output Voltage"=w174, "Test Pins.Measure Load Current"=w169, "Test Pins.Set Arbitrary Waveform"=w166) -> (w171:T17)
            n72 = Unbundle By Name(w171) -> ("Test Pins"=w170:T6)
            n73 = property on="Test Pins" class="Clust (strict)"(error in=w172, "Value"=w170) -> (error out=w167:errorcluster)  [unwired: 1 in, 1 out]
          }
          event Value Change {
            n74 = event-data() -> ("NewVal.PinName"=w177:string)  [unwired: 1 in]
            n75 = Bundle By Name(cluster=w178, "Test Pins.Measure Load Current"=w177) -> (w179:T17)
          }
          event Value Change {
            n76 = event-data() -> ("NewVal"=w182:T6, "NewVal.Set Input Voltage"=w189:string, "NewVal.Set Load Current"=w188:string, "NewVal.Measure Output Voltage"=w187:string, "NewVal.Measure Load Current"=w183:string, "NewVal.Set Arbitrary Waveform"=w181:string)  [unwired: 1 in]
            n77 = Bundle By Name(cluster=w190, "Test Pins"=w182) -> (w191:T17)
            n78 = property on="SystemSetup" class="Clust (strict)"(error in=w193) -> (error out=w192:errorcluster, "Value"=w186:T4)  [unwired: 1 in, 1 out]
            n79 = Bundle By Name(cluster=w186, "Set Input Voltage.PinName"=w189, "Power test Board.PinName"=w188, "Measure Output Voltage.PinName"=w187, "Measure Load Current.PinName"=w183, "Set Arbitrary Waveform.PinName"=w181) -> (w185:T4)
            n80 = property on="SystemSetup" class="Clust (strict)"(error in=w192, "Value"=w185) -> (error out=w184:errorcluster)  [unwired: 1 in, 1 out]
          }
          event Value Change {
            n81 = event-data() -> ("NewVal.Advance Setting"=w237:T12, "NewVal.Measure Falling Edge Slew Rate?"=w194:bool, "NewVal.Measure Rising Edge Slew Rate?"=w195:bool, "NewVal.Load Current 1 in A"=w229:dbl, "NewVal.Load Current 2 in A"=w228:dbl, "NewVal.Input Voltage in V"=w227:dbl, "NewVal.Nominal Output Voltage in V"=w226:dbl, "NewVal.Ref Voltage level for Settling Time Calc"=w225:dbl, "NewVal.% of Vnom for Settling Time Calc"=w224:dbl, "NewVal.Settling Time Calc Option"=w223:T11, "NewVal.Save Transient Graph?"=w220:bool, "NewVal.Delay - t1 in s"=w204:dbl, "NewVal.Delay - t2 in s"=w205:dbl, "NewVal.Duration of the pulse in Second"=w206:dbl, "NewVal.Save Scope Raw Data?"=w212:bool, "NewVal.Auto Scale Y-Axis?"=w211:bool, "NewVal.Shunt Resistance (Ohm)"=w209:dbl, "NewVal.Slew Rate (A/us)"=w199:dbl)  [unwired: 1 in]
            n82 = property on="Input \nVoltage 1 \n- Vin1 (V)" class="DigNum (strict)"(error in=w217, "Value"=w229) -> (error out=w230:errorcluster)  [unwired: 1 in, 1 out]
            n83 = property on="Delay - t1 (s)" class="DigNum (strict)"(error in=w217, "Value"=w204) -> (error out=w214:errorcluster)  [unwired: 1 in, 1 out]
            n84 = property on="Delay - t2 (s)" class="DigNum (strict)"(error in=w214, "Value"=w205) -> (error out=w215:errorcluster)  [unwired: 1 in, 1 out]
            n85 = property on="Input \nVoltage 2 \n- Vin2 (V)" class="DigNum (strict)"(error in=w230, "Value"=w228) -> (error out=w231:errorcluster)  [unwired: 1 in, 1 out]
            n86 = property on="Duration of the pulse (s)" class="DigNum (strict)"(error in=w215, "Value"=w206) -> (error out=w216:errorcluster)  [unwired: 1 in, 1 out]
            n87 = property on="Input Voltage (V)" class="DigNum (strict)"(error in=w231, "Value"=w227) -> (error out=w232:errorcluster)  [unwired: 1 in, 1 out]
            n88 = property on="Save Scope Raw Data?" class="Bool (strict)"(error in=w216, "Value"=w212) -> (error out=w213:errorcluster)  [unwired: 1 in, 1 out]
            n89 = property on="Nominal Output Voltage (V)" class="DigNum (strict)"(error in=w232, "Value"=w226) -> (error out=w233:errorcluster)  [unwired: 1 in, 1 out]
            n90 = property on="Auto Scale Y-Axis?" class="Bool (strict)"(error in=w213, "Value"=w211) -> (error out=w208:errorcluster)  [unwired: 1 in, 1 out]
            n91 = property on="Voltage to \nsettle above Vnom (V)" class="DigNum (strict)"(error in=w233, "Value"=w225) -> (error out=w234:errorcluster)  [unwired: 1 in, 1 out]
            n92 = property on="Shunt Resistance (Ohm)" class="DigNum (strict)"(error in=w208, "Value"=w209) -> (error out=w210:errorcluster)  [unwired: 1 in, 1 out]
            n93 = property on="Percentage \nof Vnom (%)" class="DigNum (strict)"(error in=w234, "Value"=w224) -> (error out=w238:errorcluster)  [unwired: 1 in, 1 out]
            n94 = Compound Arithmetic op=ADD(w204, w205, w206) -> (w203:dbl)
            n95 = Type Cast(type=enum32{"Item 0", "Item 1"}."Item 0" ("Settling Time Calculation"), x=w223) -> (*(type *) &x=w221:enum32{"Item 0", "Item 1"})
            n96 = Multiply(x=w203, y=5.0) -> (x*y=w201:dbl)
            n97 = property on="Settling Time Calculation" class="RadioBtnsControl (strict)"(error in=w238, "Value"=w221) -> (error out=w219:errorcluster)  [unwired: 1 in, 1 out]
            n98 = property on="Sequence Timeout" class="DigNum (strict)"(error in=w210, "Value"=w201) -> (error out=w207:errorcluster)  [unwired: 1 in, 1 out]
            n99 = Bundle By Name(cluster=w235, "Test Inputs.Advance Setting"=w237) -> (w236:T17)
            n100 = property on="Take Transient snapshot?" class="Bool (strict)"(error in=w219, "Value"=w220) -> (error out=w198:errorcluster)  [unwired: 1 in, 1 out]
            n101 = property on="Slew Rate (A/us)" class="DigNum (strict)"(error in=w207, "Value"=w199) -> (error out=w200:errorcluster)  [unwired: 1 in, 1 out]
            n102 = property on="Measure Rising Edge Slew Rate?" class="Bool (strict)"(error in=w198, "Value"=w195) -> (error out=w197:errorcluster)  [unwired: 1 in, 1 out]
            n103 = property on="Measure Falling Edge Slew Rate?" class="Bool (strict)"(error in=w197, "Value"=w194) -> (error out=w196:errorcluster)  [unwired: 1 in, 1 out]
            n104 = Merge Errors(w196, w200) -> (w218:errorcluster)
          }
          event "Tab Enum": Value Change {
            n105 = event-data() -> ("NewVal"=→"Tab Control":T1)  [unwired: 1 in]
          }
          event "Advanced Settings": Value Change {
            n106 = event-data() -> ()  [unwired: 1 in, 1 out]
            n107 = Unbundle By Name(w245) -> ("Test Inputs.Advance Setting"=w247:T12)
            n108 = call "Advance Settings UI.vi"("Advance Setting In"=w247, "error in (no error)"=w248) -> ("Advance Setting Out"=w242:T12, "error out"=w244:errorcluster)  [unwired: 12 in]
            n109 = Bundle By Name(cluster=w245, "Test Inputs.Advance Setting"=w242) -> (w246:T17)
            n110 = property on="Advance Setting" class="Clust (strict)"(error in=w244, "Value"=w242) -> (error out=w243:errorcluster)  [unwired: 1 in, 1 out]
          }
          event "Shunt Resistance (Ohm)": Value Change {
            n111 = event-data() -> ("NewVal"=w249:dbl)  [unwired: 1 in]
            n112 = property on="Shunt Resistance (Ohm)" class="DigNum (strict)"(error in=w251, "Value"=w249) -> (error out=w250:errorcluster)  [unwired: 1 in, 1 out]
          }
        }
      }
      frame "----------------- Macro ---------------" {
        # "Not used. category splitter"
      }
      frame "Macro: Initialize" {
        w261 = string[] ["Macro: GUI Start"]  # Standalone: Start the debug
        w262 = string[] ["Macro: Execute Test", "Exit"]  # Automation: Execute and stop
        # "Hidden in UI"
        # "This case decides the mode of the execution. Debug Mode: The plugin will act as a standalone GUI where user can change inputs, run test and debug the system. automation mode: The plugin will act as a flat code and go through all the test procedures and stops."
        n113 = call <userlib>:"Get Mode.vi"("Caller Information"="Caller Information", "error in (no error)"=w264) -> ("Automation(F) \\ Standalone (T)"=w260:bool, "error out"=w263:errorcluster)  [unwired: 12 in]
        n114 = Bundle By Name(cluster=w268, "Termination Monitor Info.Caller Information"="Caller Information") -> (w257:T17)
        n115 = Select(t=w261, s=w260, f=w262) -> (s? t:f=w259:string[])
        n116 = call <userlib>:"Enqueue.vi"("Queue in"=w266, "States"=w259, "Enqueue at Front?(F)"=TRUE, "error in (no error)"=w263) -> ("error out"=w267:errorcluster)  [unwired: 10 in, 1 out]
      }
      frame "Macro: Execute Test" {
        w269 = string[] ["TerminationMonitor: Start", "Test: Start", "Test: Prepare Source SMU", "Test: Prepare Load SMU", "Test: Prepare Fgen", "Test: Prepare Scope", "Test: Check on-board Size", "Test: Set Input Voltage", "Test: Calc Min Delay for Max. Ref Position", "Test: Generate Load Current Sequence", "Test: Measure Transient", "Test: Calculate Out. Voltage Threshold", "Test: Calculate Settling Time", "Test: Measure Slew Rate", "Test: Cleanup DCPower", "Test: Cleanup Scope", "Test: Cleanup Fgen", "Test: Update UI", "Test: End", "TerminationMonitor: Stop"]  # Test Procedure
        # "List the states required for the test procedure. This state will be called in both automation mode and standalone mode when requested to run the test.\nDont remove 'Test: Start' and 'Test: End'."
        n117 = call <userlib>:"Enqueue.vi"("Queue in"=w278, "States"=w269, "Enqueue at Front?(F)"=TRUE, "error in (no error)"=w279) -> ("error out"=w271:errorcluster)  [unwired: 10 in, 1 out]
        n118 = Array Size(array=w269) -> (size(s)=w273:i32)
        n119 = call "Progress Monitor.vi"("State Array []"=w269, "Option (Default: Get State Index)"=Progress_Monitor_Option."State Array Init" ("Option")) -> ()  [unwired: 13 in, 1 out]
        n120 = property on="Progress" class="Slide (strict)"(error in=w271, "Visible"=TRUE, "Scale.Maximum"=w273, "Value"=0 ("Progress")) -> (error out=w270:errorcluster)  [unwired: 1 in, 1 out]
      }
      frame "Macro: GUI Start" {
        # "Initialize the data cluster for the standalone mode and register for the event from caller.\nDon't remove 'GUI: Initialize Data' and 'GUI: Register Event'."
        n121 = call <userlib>:"Enqueue.vi"("Queue in"=w283, "States"=string[] ["GUI: Initialize Data", "GUI: Register Event"], "Enqueue at Front?(F)"=TRUE, "error in (no error)"=w285) -> ("error out"=w286:errorcluster)  [unwired: 10 in, 1 out]
      }
      frame "Macro: GUI Stop" {
        # "Cleanups the standalone mode and stop the execution.\nDon't remove 'GUI: Unregister Event', 'GUI: Cleanup Data' and 'Exit'."
        n122 = call <userlib>:"Enqueue.vi"("Queue in"=w290, "States"=string[] ["GUI: Unregister Event", "GUI: Cleanup Data", "Exit"], "Enqueue at Front?(F)"=TRUE, "error in (no error)"=w292) -> ("error out"=w293:errorcluster)  [unwired: 10 in, 1 out]
      }
      frame "--------------- GUI Mode-----------------" {
        # "Not used. category splitter"
      }
      frame "GUI: Initialize Data" {
        w300 = TRUE ("Visible")
        w326 = T1."Station Setup" ("Tab Enum")
        w329 = string[][] []  # Test Results[][]
        w338 = T15 {"Measured Output Voltage"={"x-axis"=[], "wfm"=[]}, "Measured Load Current"={"x-axis"=[], "wfm"=[]}, "Actual Sample Rate in S/s"=0.0, "First Edge - Settling Time in s"=0.0, "Second Edge - Settling Time in s"=0.0, "Rising Edge - Measured Slew Rate (A/us)"=0.0, "Falling Edge - Measured Slew Rate (A/us)"=0.0}  # Test Results
        # "Add the front panel controls terminal here and connect them to the bundle structure, So they will be available through data cluster in every case. If the controls and indicators are added to the 'Test Inputs' & 'Test Results' cluster then they are already available in the data cluster since they are typedefs."
        n123 = property on="Run" class="Bool (strict)"(error in=w332, "DisabledEnum"=T19."Enabled" ("Disabled")) -> (error out=w335:errorcluster)  [unwired: 1 in, 1 out]
        n124 = local write "Tab Enum"(w326) -> ()
        n125 = local write "Tab Control"(w326) -> ()
        n126 = property on="Terminate" class="Bool (strict)"(error in=w335, "DisabledEnum"=T19."Disabled and Grayed Out" ("Disabled")) -> (error out=w331:errorcluster)  [unwired: 1 in, 1 out]
        n127 = property on="Progress" class="Slide (strict)"(error in=w331, "Visible"=FALSE) -> (error out=w299:errorcluster)  [unwired: 1 in, 1 out]
        n128 = property on="Shunt Resistance (Ohm)" class="DigNum (strict)"(error in=w299, "Visible"=w300) -> (error out=w301:errorcluster)  [unwired: 1 in, 1 out]
        n129 = Bundle By Name(cluster=w337, "Test Pins"="Test Pins", "Test Inputs"="Test Inputs", "Test Results"=w338, "Test Results[][]"=w329, "Logger Folder Path"="DataLogPath") -> (w324:T17)
        n130 = property on="Shunt Resistance Info" class="Ring (strict)"(error in=w301, "Visible"=w300) -> (error out=w298:errorcluster)  [unwired: 1 in, 1 out]
        n131 = control-ref of="Settling Time Calculation"() -> (w309:refnum<vi>)
        n132 = control-ref of="Auto Scale Y-Axis?"() -> (w308:refnum<vi>)
        n133 = control-ref of="Save Scope Raw Data?"() -> (w307:refnum<vi>)
        n134 = control-ref of="Take Transient snapshot?"() -> (w306:refnum<vi>)
        n135 = control-ref of="Advanced Settings"() -> (w305:refnum<vi>)
        n136 = control-ref of="SystemSetup"() -> (w322:refnum<vi>)
        n137 = control-ref of="Sequence Timeout"() -> (w304:refnum<vi>)
        n138 = control-ref of="First Edge - Settling Time (s)"() -> (w303:refnum<vi>)
        n139 = control-ref of="Second Edge - Settling Time (s)"() -> (w302:refnum<vi>)
        n140 = control-ref of="Shunt Resistance (Ohm)"() -> (w320:refnum<vi>)
        n141 = control-ref of="Input Voltage (V)"() -> (w318:refnum<vi>)
        n142 = control-ref of="Load Current 1 - Iload1 (A)"() -> (w317:refnum<vi>)
        n143 = control-ref of="Load Current 2 - Iload2 (A)"() -> (w316:refnum<vi>)
        n144 = control-ref of="Delay - t1 (s)"() -> (w315:refnum<vi>)
        n145 = control-ref of="Duration of the pulse (s)"() -> (w314:refnum<vi>)
        n146 = control-ref of="Delay - t2 (s)"() -> (w313:refnum<vi>)
        n147 = control-ref of="Nominal Output Voltage (V)"() -> (w312:refnum<vi>)
        n148 = control-ref of="Voltage to settle above Vnom (V)"() -> (w311:refnum<vi>)
        n149 = control-ref of="Percentage of Vnom (%)"() -> (w310:refnum<vi>)
        n150 = control-ref of="Shunt Resistance Info"() -> (w319:refnum<vi>)
        n151 = Build Array(w322, w320, w319, w318, w317, w316, w315, w314, w313, w312, w311, w310, w309, w308, w307, w306, w305, w304, w303, w302) -> (w321:refnum<vi>[])
        n152 = Bundle By Name(cluster=w324, "UI Ctls"=w321) -> (w323:T17)
      }
      frame "GUI: Register Event" {
        # "Hidden in UI"
        # "Register for the events from caller."
        n153 = register-events(error in=w343, "Caller Events") -> (reference out=w340:refnum<event-registration>, error out=w341:errorcluster)  [unwired: 1 in]
      }
      frame "GUI: Unregister Event" {
        n154 = Unregister For Events(event registration refnum=w344, error in=w347) -> (error out=w345:errorcluster)
      }
      frame "GUI: Cleanup Data" {
        # "Cleanup the reference or other resources before exiting"
      }
      frame "GUI: Set Busy" {
        n155 = call "Progress Monitor.vi"("State"=w351) -> ("State Array Index"=w354:i32)  [unwired: 14 in]
        n156 = property on="Progress" class="Slide (strict)"(error in=w352, "Value"=w354) -> (error out=w353:errorcluster)  [unwired: 1 in, 1 out]
        n157 = Unbundle By Name(w355) -> ("UI Ctls"=w360:refnum<vi>[])
        n158 = for {
          tunnel: [w365] -> w361 mode=indexing
          tunnel: w353 -> [w366]
          tunnel: w360 -> [w364] mode=indexing
          tunnel: T19."Disabled and Grayed Out" ("Disabled") -> [w363]
          n159 = property class="Ctl"(reference=w364, error in=w366, "DisabledEnum"=w363) -> (error out=w365:errorcluster)  [unwired: 1 out]
        }
        n160 = Merge Errors(w361) -> (w358:errorcluster)
        n161 = call "Defer Front Panel.vi"("Defer Front Panel?"=TRUE, "error in"=w358) -> ("error out"=w356:errorcluster)  [unwired: 13 in]
      }
      frame "GUI: Unset Busy" {
        n162 = call "Progress Monitor.vi"("State"=w367) -> ("State Array Index"=w368:i32)  [unwired: 14 in]
        n163 = property on="Progress" class="Slide (strict)"(error in=w369, "Value"=w368) -> (error out=w370:errorcluster)  [unwired: 1 in, 1 out]
        n164 = Unbundle By Name(w371) -> ("UI Ctls"=w376:refnum<vi>[])
        n165 = for {
          tunnel: [w381] -> w377 mode=indexing
          tunnel: w370 -> [w382]
          tunnel: w376 -> [w380] mode=indexing
          tunnel: T19."Enabled" ("Disabled") -> [w379]
          n166 = property class="Ctl"(reference=w380, error in=w382, "DisabledEnum"=w379) -> (error out=w381:errorcluster)  [unwired: 1 out]
        }
        n167 = Merge Errors(w377) -> (w373:errorcluster)
        n168 = call "Defer Front Panel.vi"("Defer Front Panel?"=FALSE, "error in"=w373) -> ("error out"=w372:errorcluster)  [unwired: 13 in]
      }
      frame "GUI: Update Sequence Timeout" {
        # "Multiply by 5 to have sufficient timeout"
        n169 = Unbundle By Name(w391) -> ("Test Inputs.Delay - t1 in s"=w390:dbl, "Test Inputs.Delay - t2 in s"=w389:dbl, "Test Inputs.Duration of the pulse in Second"=w388:dbl)
        n170 = Compound Arithmetic op=ADD(w390, w389, w388) -> (w383:dbl)
        n171 = Multiply(x=w383, y=5.0) -> (x*y=w387:dbl)
        n172 = property on="Sequence Timeout" class="DigNum (strict)"(error in=w384, "Value"=w387) -> (error out=w385:errorcluster)  [unwired: 1 in, 1 out]
      }
      frame "GUI: Get Logger File Path" {
        n173 = Unbundle By Name(w393) -> ("Logger Folder Path"=w400:path)
        n174 = call <vilib>:"Check if File or Folder Exists.vi"("error in (no error)"=w396, "path"=w400) -> ("error out"=w399:errorcluster, "file or folder exists?"=w398:bool, "dup path"=w397:path)  [unwired: 7 in]
        n175 = case shown="True" w398 {
          tunnel: [w403 w412] -> w395
          tunnel: w399 -> [w403 w415]
          tunnel: w393 -> [w402 w419]
          tunnel: [w402 w418] -> w394
          tunnel: w397 -> [_ w414]
          frame False {
          }
          frame True {
            n176 = Strip Path(path=w414) -> (name=w406:string)  [unwired: 1 out]
            n177 = call "Get Unique Name.vi"() -> ("date"=w413:string, "Unique String"=w405:string)  [unwired: 14 in]
            n178 = Concatenate Strings(w406, w413) -> (w409:string)
            n179 = Concatenate Strings(w406, w405) -> (w404:string)
            n180 = Concatenate Strings(w409, "\\" ("string"), w404) -> (w416:string)
            n181 = Build Path(base path=w414, name or relative path=w416) -> (appended path=w411:path)
            n182 = call <vilib>:"Create Directory Recursive.vi"("error in (no error)"=w415, "directory"=w411) -> ("error out"=w412:errorcluster, "directory copy"=w408:path)  [unwired: 3 in, 1 out]
            n183 = Build Path(base path=w408, name or relative path=w404) -> (appended path=w407:path)
            n184 = Bundle By Name(cluster=w419, "Valid Logger Path?"=TRUE ("Valid Logger path?"), "Logger File Path"=w407) -> (w418:T17)
          }
        }
      }
      frame "GUI: Log" {
        n185 = Unbundle By Name(w427) -> ("Test Inputs.Save Scope Raw Data?"=w420:bool, "Valid Logger Path?"=w421:bool, "Test Inputs"=w423:T10, "Test Results"=w424:T15, "Logger File Path"=w422:path)
        n186 = case shown="True" w421 {
          tunnel: [w429 w435] -> w426
          tunnel: w425 -> [w429 w434]
          tunnel: w424 -> [_ w433]
          tunnel: w423 -> [_ w432]
          tunnel: w422 -> [_ w431]
          tunnel: w420 -> [_ w430]
          frame False {
          }
          frame True {
            n187 = call "Log Data.vi"("Test Inputs"=w432, "Save Scope Raw Data?"=w430, "Test Results"=w433, "DataLogger File Path"=w431, "error in (no error)"=w434) -> ("error out"=w435:errorcluster)  [unwired: 10 in]
          }
        }
      }
      frame "GUI: Update Graph Scale" {
        w449 = u32 1 ("Active Plot")
        w450 = u32 0 ("Active Plot")
        # "Placing plot legend inside graph in top right"
        n188 = Unbundle By Name(w452) -> ("Test Inputs.Auto Scale Y-Axis?"=w451:bool)
        n189 = control-ref of="Load Transient"() -> (w437:refnum<vi>)
        n190 = property class="XYGraph (strict)"(reference=w437, error in=w438) -> (reference out=w446:refnum<vi>, error out=w447:errorcluster, "Left"=w445:i32, "Top"=w444:i32)
        n191 = Add(x=w444, y=11) -> (x+y=w440:i32)
        n192 = Add(x=w445, y=418) -> (x+y=w441:i32)
        n193 = property on="Property Node" class="XYGraph (strict)"(reference=w446, error in=w447, "Active Plot"=w450, "Plot.YScaleIdx"=w450, "Active Plot"=w449, "Plot.YScaleIdx"=w449, "LegLeft"=w441, "LegTop"=w440) -> (reference out=w439:refnum<vi>, error out=w448:errorcluster)
        n194 = case shown="True" w451 {
          tunnel: [w454 w457] -> w436
          tunnel: w448 -> [w454 w456]
          tunnel: w439 -> [_ w455]
          frame False {
          }
          frame True {
            n195 = call "Two Plot XY Graph Auto Scale.vi"("Two Plot XY Graph Ref In"=w455, "error in (no error)"=w456) -> ("error out"=w457:errorcluster)  [unwired: 12 in, 1 out]
          }
        }
      }
      frame "GUI: Log Waveform Snapshot" {
        n196 = Unbundle By Name(w458) -> ("Test Inputs.Save Transient Graph?"=w464:bool, "Valid Logger Path?"=w462:bool, "Logger File Path"=w461:path)
        n197 = And(x=w464, y=w462) -> (x .and. y?=w463:bool)
        n198 = case shown="True" w463 {
          tunnel: w459 -> [w466 w468]
          tunnel: [w466 w467] -> w460
          tunnel: w461 -> [_ w469]
          frame False {
          }
          frame True {
            w475 = T21 {"Major Color"=14737632, "Minor Color"=15987699} ("Y Scale.Grid Colors")
            w476 = T21 {"Major Color"=16777216, "Minor Color"=16777216} ("Y Scale.Grid Colors")
            n199 = control-ref of="Load Transient"() -> (w470:refnum<vi>)
            n200 = Path To String(path=w469) -> (string=w487:string)
            n201 = property class="XYGraph (strict)"(reference=w470, error in=w468, "ActYScl"=0 ("Active Y Scale"), "YScale.GridColors"=w476, "ActYScl"=1 ("Active Y Scale"), "YScale.GridColors"=w476) -> (reference out=w479:refnum<vi>, error out=w480:errorcluster)
            n202 = Concatenate Strings(w487, "_Waveform" ("string"), ".bmp" ("format string")) -> (w488:string)
            n203 = String To Path(string=w488) -> (path=w486:path)
            n204 = invoke class="XYGraph (strict)" method="Export Image"(reference=w479, error in=w480, "FileType"=enum32{"BMP", "EPS", "EMF", "PICT"}."BMP" ("File Type"), "Target"=enum32{"File", "Clipboard"}."File", "Path"=w486, "HideGrid"=TRUE ("Hide Grid")) -> (reference out=w471:refnum<vi>, error out=w472:errorcluster)  [unwired: 2 in, 6 out]
            n205 = property class="XYGraph (strict)"(reference=w471, error in=w472, "ActYScl"=0 ("Active Y Scale"), "YScale.GridColors"=w475, "ActYScl"=1 ("Active Y Scale"), "YScale.GridColors"=w475) -> (error out=w467:errorcluster)  [unwired: 1 out]
          }
        }
      }
      frame "GUI: Start Test" {
        n206 = property on="Run" class="Bool (strict)"(error in=w491, "DisabledEnum"=T19."Disabled and Grayed Out" ("Disabled")) -> (error out=w496:errorcluster)  [unwired: 1 in, 1 out]
        n207 = property on="Terminate" class="Bool (strict)"(error in=w496, "DisabledEnum"=T19."Enabled" ("Disabled")) -> (error out=w494:errorcluster)  [unwired: 1 in, 1 out]
        n208 = property on="Progress" class="Slide (strict)"(error in=w494, "Visible"=TRUE, "Value"=0 ("Progress")) -> (error out=w492:errorcluster)  [unwired: 1 in, 1 out]
      }
      frame "GUI: End Test" {
        n209 = property on="Run" class="Bool (strict)"(error in=w500, "Value"=FALSE ("Run"), "DisabledEnum"=T19."Enabled" ("Disabled")) -> (error out=w506:errorcluster)  [unwired: 1 in, 1 out]
        n210 = property on="Terminate" class="Bool (strict)"(error in=w506, "DisabledEnum"=T19."Disabled and Grayed Out" ("Disabled")) -> (error out=w505:errorcluster)  [unwired: 1 in, 1 out]
        n211 = property on="Progress" class="Slide (strict)"(error in=w505, "Visible"=FALSE) -> (error out=w499:errorcluster)  [unwired: 1 in, 1 out]
      }
      frame "------------ TerminationMonitor -----------" {
        # "Not used. category splitter"
      }
      frame "TerminationMonitor: Start" {
        # "Termination Monitor monitors the execution of the caller. Use Termination Monitor Status to get the termination status. If the caller is terminating, stop the test procedure, cleanup and stop."
        n212 = Unbundle By Name(w514) -> ("Termination Monitor Info.Caller Information"=w513:T7)
        n213 = call <userlib>:"Termination Monitor Start.vi"("Caller Information"=w513, "error in (no error)"=w516) -> ("Termination Monitor Info out"=w512:T16, "error out"=w517:errorcluster)  [unwired: 12 in]
        n214 = Bundle By Name(cluster=w514, "Termination Monitor Info"=w512) -> (w515:T17)
      }
      frame "TerminationMonitor: Stop" {
        n215 = Unbundle By Name(w521) -> ("Termination Monitor Info"=w520:T16)
        n216 = call <userlib>:"Termination Monitor Stop.vi"("Status Info in"=w520, "error in (no error)"=w523) -> ("Status Info out"=w519:T16, "error out"=w524:errorcluster)  [unwired: 12 in]
        n217 = Bundle By Name(cluster=w521, "Termination Monitor Info"=w519) -> (w522:T17)
      }
      frame "------------ Automation Mode -----------" {
        # "Not used. category splitter"
      }
      frame "Test: Start" {
        # "Reinitialize/Reset/Update the data from the UI to the data cluster so that the data will be considered for the test procedure.\nReset the Test Results."
        n218 = call "Progress Monitor.vi"("State"=w529) -> ("State Array Index"=w532:i32)  [unwired: 14 in]
        n219 = property on="Progress" class="Slide (strict)"(error in=w530, "Value"=w532) -> (error out=w531:errorcluster)  [unwired: 1 in, 1 out]
        n220 = local read "DataLogPath"() -> (w533:path)
        n221 = local read "Test Inputs"() -> (w544:T10)
        n222 = local read "Test Pins"() -> (w534:T6)
        n223 = property on="Run" class="Bool (strict)"(error in=w531, "DisabledEnum"=T19."Disabled and Grayed Out" ("Disabled")) -> (error out=w540:errorcluster)  [unwired: 1 in, 1 out]
        n224 = Bundle By Name(cluster=w545, "Test Pins"=w534, "Test Inputs"=w544, "Test Results"=T15 {"Measured Output Voltage"={"x-axis"=[], "wfm"=[]}, "Measured Load Current"={"x-axis"=[], "wfm"=[]}, "Actual Sample Rate in S/s"=0.0, "First Edge - Settling Time in s"=0.0, "Second Edge - Settling Time in s"=0.0, "Rising Edge - Measured Slew Rate (A/us)"=0.0, "Falling Edge - Measured Slew Rate (A/us)"=0.0}, "Logger Folder Path"=w533) -> (w535:T17)
        n225 = property on="Terminate" class="Bool (strict)"(error in=w540, "DisabledEnum"=T19."Enabled" ("Disabled")) -> (error out=w537:errorcluster)  [unwired: 1 in, 1 out]
        n226 = property on="Progress" class="Slide (strict)"(error in=w537, "Visible"=FALSE) -> (error out=w536:errorcluster)  [unwired: 1 in, 1 out]
      }
      frame "Test: Prepare Source SMU" {
        n227 = call "Progress Monitor.vi"("State"=w549) -> ("State Array Index"=w552:i32)  [unwired: 14 in]
        n228 = property on="Progress" class="Slide (strict)"(error in=w550, "Value"=w552) -> (error out=w551:errorcluster)  [unwired: 1 in, 1 out]
        n229 = Unbundle By Name(w553) -> ("Test Pins.Set Input Voltage"=w546:string, "Test Inputs.Input Voltage in V"=w547:dbl)
        n230 = call "Prepare Source.vi"("Set Vin"=w546, "Initial Voltage Level (V)"=w547, "error in (no error)"=w551) -> ("error out"=w548:errorcluster)  [unwired: 12 in]
      }
      frame "Test: Prepare Load SMU" {
        w581 = T22 1030 items=["Source Complete Event"=1030, "Measure Complete Event"=1031, "Sequence Iteration Complete Event"=1032, "Sequence Engine Done Event"=1033, "Pulse Complete Event"=1051, "Ready For Pulse Trigger Event"=1052] ("event")
        w572 = TRUE  # output enabled
        w566 = T23 1006 items=["DC Voltage"=1006, "DC Current"=1007, "Pulse Voltage"=1049, "Pulse Current"=1050] ("output function")
        w569 = T24 1020 items=["Single Point"=1020, "Sequence"=1021] ("source mode")
        n231 = call "Progress Monitor.vi"("State"=w582) -> ("State Array Index"=w584:i32)  [unwired: 14 in]
        n232 = property on="Progress" class="Slide (strict)"(error in=w583, "Value"=w584) -> (error out=w563:errorcluster)  [unwired: 1 in, 1 out]
        n233 = Unbundle By Name(w585) -> ("Test Inputs.Advance Setting.Prepare.Power Test Board.Current Limit (A)"=w556:dbl, "Test Inputs.Advance Setting.Prepare.Power Test Board.Voltage Level (V)"=w560:dbl, "Test Pins.Set Load Current"=w561:string)
        n234 = Absolute Value(x=w556) -> (abs(x)=w555:dbl)
        n235 = call "Pin Name to Reference.vim"("Pin Name"=w561, "type"=refnum<k15> refnum ("instrument handle"), "error in (no error)"=w563) -> ("Reference"=w578:refnum<k15>, "error out"=w577:errorcluster)  [unwired: 7 in, 4 out]
        n236 = call <instrlib>:"niDCPower Abort.vi"("error in (no error)"=w577, "instrument handle"=w578) -> ("error out"=w565:errorcluster, "instrument handle out"=w564:refnum<k15>)  [unwired: 8 in]
        n237 = call <instrlib>:"niDCPower Configure Source Mode With Channels.vi"("error in (no error)"=w565, "source mode"=w569, "instrument handle"=w564) -> ("error out"=w567:errorcluster, "instrument handle out"=w568:refnum<k15>)  [unwired: 7 in]
        n238 = call <instrlib>:"niDCPower Configure Output Function.vi"("error in (no error)"=w567, "output function"=w566, "instrument handle"=w568) -> ("error out"=w570:errorcluster, "instrument handle out"=w571:refnum<k15>)  [unwired: 7 in]
        n239 = call <instrlib>:"niDCPower Configure Voltage Level.vi"("error in (no error)"=w570, "voltage level"=w560, "instrument handle"=w571) -> ("error out"=w573:errorcluster, "instrument handle out"=w558:refnum<k15>)  [unwired: 7 in]
        n240 = call <instrlib>:"niDCPower Configure Current Limit.vi"("error in (no error)"=w573, "current limit"=w555, "instrument handle"=w558) -> ("error out"=w559:errorcluster, "instrument handle out"=w557:refnum<k15>)  [unwired: 7 in]
        n241 = call <instrlib>:"niDCPower Configure Output Enabled.vi"("error in (no error)"=w559, "output enabled"=w572, "instrument handle"=w557) -> ("error out"=w574:errorcluster, "instrument handle out"=w575:refnum<k15>)  [unwired: 7 in]
        n242 = call <instrlib>:"niDCPower Initiate.vi"("error in (no error)"=w574, "instrument handle"=w575) -> ("error out"=w579:errorcluster, "instrument handle out"=w580:refnum<k15>)  [unwired: 8 in]
        n243 = call <instrlib>:"niDCPower Wait For Event With Channels.vi"("error in (no error)"=w579, "event"=w581, "instrument handle"=w580) -> ("error out"=w562:errorcluster)  [unwired: 7 in, 1 out]
      }
      frame "Test: Prepare Scope" {
        # "Set sampling rate"
        # "Aborting prev acquisition"
        n244 = Unbundle By Name(w611) -> ("Test Pins.Measure Load Current"=w610:string, "Test Pins.Measure Output Voltage"=w618:string)
        n245 = call "Progress Monitor.vi"("State"=w613) -> ("State Array Index"=w616:i32)  [unwired: 14 in]
        n246 = property on="Progress" class="Slide (strict)"(error in=w614, "Value"=w616) -> (error out=w615:errorcluster)  [unwired: 1 in, 1 out]
        n247 = call "Pin Name to Reference.vim"("Pin Name"=w618, "type"=refnum<k15> refnum ("instrument handle"), "error in (no error)"=w615) -> ("Reference"=w598:refnum<k15>, "Channel"=w596:string, "error out"=w606:errorcluster)  [unwired: 7 in, 3 out]
        n248 = call <instrlib>:"niScope Abort.vi"("instrument handle"=w598, "error in"=w606) -> ("instrument handle out"=w597:refnum<k15>, "error out"=w599:errorcluster)  [unwired: 12 in]
        n249 = property class="niScope"(reference=w597, error in=w599, "Active Channel"=w596, "Channel Enabled"=TRUE ("Vertical:Channel Enabled")) -> (error out=w602:errorcluster, "Vertical Coupling"=w608:i32)  [unwired: 1 out]
        n250 = call "Pin Name to Reference.vim"("Pin Name"=w610, "type"=refnum<k15> refnum ("instrument handle"), "error in (no error)"=w602) -> ("Reference"=w592:refnum<k15>, "Channel"=w587:string, "error out"=w593:errorcluster)  [unwired: 7 in, 3 out]
        n251 = Build Array(w596, w587) -> (w588:string[])
        n252 = property class="niScope"(reference=w592, error in=w593, "Active Channel"=w587, "Channel Enabled"=TRUE ("Vertical:Channel Enabled")) -> (reference out=w600:refnum<k15>, error out=w601:errorcluster)
        n253 = Array To Spreadsheet String(delimiter (Tab)=",", array=w588, 3:"" ("format string")) -> (spreadsheet string=w609:string)
        n254 = property class="niScope"(reference=w600, error in=w601) -> (reference out=w603:refnum<k15>, error out=w604:errorcluster, "Actual Sample Rate"=w595:dbl)
        n255 = property class="niScope"(reference=w603, error in=w604, "Min Sample Rate"=w595) -> (error out=w617:errorcluster)  [unwired: 1 out]
        n256 = Bundle By Name(cluster=w611, "Scope Channels"=w609, "Output Voltage Coupling"=w608) -> (w612:T17)
      }
      frame "Test: Prepare Fgen" {
        w624 = T25 2 items=["Standard Function", "Frequency List", "Arbitrary Waveform", "Arbitrary Sequence", "Script"] ("Output Mode (default: 0=Standard Function)")
        w630 = T26 0 items=["Single", "Continuous", "Stepped", "Burst"] ("Trigger Mode")
        n257 = Unbundle By Name(w637) -> ("Test Inputs.Advance Setting.Prepare.Fgen.Sample Rate (Sample/s)"=w623:dbl, "Test Pins.Set Arbitrary Waveform"=w633:string)
        n258 = call "Pin Name to Reference.vim"("Pin Name"=w633, "type"=refnum<k15> refnum ("instrument handle"), "error in (no error)"=w634) -> ("Reference"=w622:refnum<k15>, "error out"=w635:errorcluster)  [unwired: 7 in, 4 out]
        n259 = call <instrlib>:"niFgen Abort Generation.vi"("error in (no error)"=w635, "Instrument Handle"=w622) -> ("error out"=w625:errorcluster, "Instrument Handle Out"=w621:refnum<k15>)  [unwired: 8 in]
        n260 = call <instrlib>:"niFgen Configure Output Mode.vi"("error in (no error)"=w625, "Output Mode (default: 0=Standard Function)"=w624, "Instrument Handle"=w621) -> ("error out"=w628:errorcluster, "Instrument Handle Out"=w629:refnum<k15>)  [unwired: 6 in]
        n261 = call <instrlib>:"niFgen Configure Trigger Mode.vi"("error in (no error)"=w628, "Trigger Mode (default: 1=continuous)"=w630, "Instrument Handle"=w629) -> ("error out"=w626:errorcluster, "Instrument Handle Out"=w627:refnum<k15>)  [unwired: 7 in]
        n262 = call <instrlib>:"niFgen Clear Arbitrary Memory.vi"("error in (no error)"=w626, "Instrument Handle"=w627) -> ("error out"=w631:errorcluster, "Instrument Handle Out"=w632:refnum<k15>)  [unwired: 8 in]
        n263 = call <instrlib>:"niFgen Set Sample Rate.vi"("error in (no error)"=w631, "Sample Rate (Samp/s)"=w623, "Instrument Handle"=w632) -> ("error out"=w620:errorcluster)  [unwired: 7 in, 1 out]
      }
      frame "Test: Check on-board Size" {
        # "A/s conversion"
        # "Acquired Time = Time 1+ Duration of pulse +Time 2 + [2 * slope time]"
        n264 = Unbundle By Name(w659) -> ("Test Inputs.Delay - t1 in s"=w656:dbl, "Test Inputs.Delay - t2 in s"=w655:dbl, "Test Inputs.Duration of the pulse in Second"=w654:dbl, "Test Inputs.Load Current 1 in A"=w650:dbl, "Test Inputs.Load Current 2 in A"=w649:dbl, "Test Inputs.Slew Rate (A/us)"=w646:dbl, "Test Pins.Measure Output Voltage"=w652:string)
        n265 = Subtract(x=w650, y=w649) -> (x-y=w651:dbl)
        n266 = Absolute Value(x=w651) -> (abs(x)=w648:dbl)
        n267 = Multiply(x=w646, y=1000000.0) -> (x*y=w647:dbl)
        n268 = Divide(x=w648, y=w647) -> (x/y=w644:dbl)
        n269 = Compound Arithmetic op=ADD(w656, w655, w654, w644, w644) -> (w643:dbl)
        n270 = call "Check Scope on-board memory.vi"("Scope"=w652, "Acquisition Time"=w643, "error in (no error)"=w657) -> ("IVI Refnum out"=w641:refnum<k15>, "Required Record Length"=w640:i32, "Maximum Record Length"=w639:i32, "Insufficient Memory?"=w653:bool, "error out"=w642:errorcluster)  [unwired: 8 in]
        n271 = case shown="True" w653 {
          tunnel: w642 -> [w665 w669]
          tunnel: [w664 w668] -> w658
          tunnel: w641 -> [w663 _]
          tunnel: w640 -> [w662 w667]
          tunnel: w639 -> [_ w666]
          frame False {
            # "Valid memory"
            n272 = property class="niScope"(reference=w663, error in=w665, "Min Number of Points"=w662) -> (error out=w664:errorcluster)  [unwired: 1 out]
          }
          frame True {
            # "Show error"
            n273 = call "Error 6005.vi"("Requested Record Length"=w667, "Maximum Record Length"=w666, "error in (no error)"=w669) -> ("error out"=w668:errorcluster)  [unwired: 12 in]
          }
        }
        n274 = Bundle By Name(cluster=w659, "Scope Acquired time(s)"=w643, "Insufficient memory?"=w653) -> (w660:T17)
      }
      frame "Test: Set Input Voltage" {
        n275 = call "Progress Monitor.vi"("State"=w673) -> ("State Array Index"=w676:i32)  [unwired: 14 in]
        n276 = property on="Progress" class="Slide (strict)"(error in=w674, "Value"=w676) -> (error out=w675:errorcluster)  [unwired: 1 in, 1 out]
        n277 = Unbundle By Name(w677) -> ("Test Pins.Set Input Voltage"=w670:string, "Test Inputs.Input Voltage in V"=w671:dbl)
        n278 = call "Set Source.vi"("Set Vin"=w670, "Vin in V"=w671, "error in (no error)"=w675) -> ("error out"=w672:errorcluster)  [unwired: 12 in]
      }
      frame "Test: Calc Min Delay for Max. Ref Position" {
        n279 = call "Progress Monitor.vi"("State"=w680) -> ("State Array Index"=w683:i32)  [unwired: 14 in]
        n280 = property on="Progress" class="Slide (strict)"(error in=w681, "Value"=w683) -> (error out=w682:errorcluster)  [unwired: 1 in, 1 out]
        n281 = Unbundle By Name(w684) -> ("Insufficient memory?"=w679:bool, "Test Pins.Measure Output Voltage"=w687:string)
        n282 = disable-structure shown="Enabled" {
          disable-tunnel: [w694 _] -> w688
          disable-tunnel: w687 -> [w693 _]
          disable-tunnel: [w692 _] -> w686
          disable-tunnel: w682 -> [w691 _]
          disable-tunnel: w679 -> [w690 _]
          frame Enabled {
            n283 = case shown="False" w690 {
              tunnel: [w712 w713] -> w694
              tunnel: w693 -> [w711 _]
              tunnel: [w710 _] -> w692
              tunnel: w691 -> [w709 w713]
              frame False {
                # "Reference Position % of Total Aqusition Time"
                # "in milliseconds"
                # "Total Acquisition Time"
                # "Sufficient Buffer and on-board memory and has valid sequence"
                n284 = call "Pin Name to Reference.vim"("Pin Name"=w711, "type"=refnum<k15> refnum ("instrument handle"), "error in (no error)"=w709) -> ("Reference"=w706:refnum<k15>, "error out"=w707:errorcluster)  [unwired: 7 in, 4 out]
                n285 = property class="niScope"(reference=w706, error in=w707) -> (error out=w712:errorcluster, "Reference Position"=w695:dbl, "Min Number of Points"=w696:i32, "Actual Sample Rate"=w705:dbl)  [unwired: 1 out]
                n286 = Reciprocal(x=w705) -> (1/x=w704:dbl)
                n287 = To Double Precision Float(number=w696) -> (double precision float=w703:dbl)
                n288 = Multiply(x=w703, y=w704) -> (x*y=w702:dbl)
                n289 = Divide(x=w695, y=100.0) -> (x/y=w701:dbl)
                n290 = Multiply(x=w701, y=w702) -> (x*y=w699:dbl)
                n291 = Multiply(x=w699, y=1000.0) -> (x*y=w697:dbl)
                n292 = To Unsigned Long Integer(number=w697) -> (unsigned 32bit integer=w710:u32)
              }
              frame True {
                # "Insufficient buffer and on-board memory"
              }
            }
          }
          frame Disabled {
          }
        }
        n293 = Bundle By Name(cluster=w684, "Min delay for Reference Position"=w686) -> (w685:T17)
      }
      frame "Test: Generate Load Current Sequence" {
        n294 = call "Progress Monitor.vi"("State"=w728) -> ("State Array Index"=w730:i32)  [unwired: 14 in]
        n295 = property on="Progress" class="Slide (strict)"(error in=w729, "Value"=w730) -> (error out=w727:errorcluster)  [unwired: 1 in, 1 out]
        n296 = Unbundle By Name(w731) -> ("Test Inputs.Advance Setting.Prepare.Sense Resistance (Ohm)"=w716:dbl, "Test Inputs.Delay - t1 in s"=w717:dbl, "Test Inputs.Duration of the pulse in Second"=w718:dbl, "Test Inputs.Delay - t2 in s"=w719:dbl, "Test Inputs.Load Current 1 in A"=w720:dbl, "Test Inputs.Load Current 2 in A"=w721:dbl, "Test Inputs.Slew Rate (A/us)"=w722:dbl, "Test Inputs.Advance Setting.Stimulus And Measure.Fgen.Offset (V)"=w715:dbl, "Test Pins.Set Arbitrary Waveform"=w725:string, "Min delay for Reference Position"=w724:u32, "Test Pins.Measure Output Voltage"=w726:string, "Insufficient memory?"=w723:bool)
        n297 = case shown="False" w723 {
          tunnel: w727 -> [w754 w756]
          tunnel: w726 -> [w753 _]
          tunnel: w725 -> [w750 _]
          tunnel: [w745 w756] -> w714
          tunnel: w724 -> [w746 _]
          tunnel: w722 -> [w741 _]
          tunnel: w721 -> [w740 _]
          tunnel: w720 -> [w739 _]
          tunnel: w719 -> [w738 _]
          tunnel: w718 -> [w737 _]
          tunnel: w717 -> [w736 _]
          tunnel: w716 -> [w735 _]
          tunnel: w715 -> [w734 _]
          frame False {
            # "Sufficient buffer and on-board memory and has valid sequence"
            n298 = call "Pin Name to Reference.vim"("Pin Name"=w753, "type"=refnum<k15> refnum ("instrument handle"), "error in (no error)"=w754) -> ("Reference"=w751:refnum<k15>, "error out"=w752:errorcluster)  [unwired: 7 in, 4 out]
            n299 = call <instrlib>:"niScope Initiate Acquisition.vi"("instrument handle"=w751, "error in"=w752) -> ("error out"=w748:errorcluster)  [unwired: 12 in, 1 out]
            n300 = call "Stall Data Flow.vim"("value in"=w748, "milliseconds to wait"=w746) -> ("value out"=w747:errorcluster)  [unwired: 1 out]
            n301 = call "Pin Name to Reference.vim"("Pin Name"=w750, "type"=refnum<k15> refnum ("instrument handle"), "error in (no error)"=w747) -> ("Reference"=w744:refnum<k15>, "error out"=w733:errorcluster)  [unwired: 7 in, 4 out]
            n302 = Bundle By Name(cluster=T20 {"Delay - t1 (s)"=10.0, "Duration of the pulse (s)"=10.0, "Delay - t2 (s)"=10.0, "Load Current 1 - Iload1 (A)"=1.0, "Load Current 2 - Iload2 (A)"=0.0, "Slew rate A/us"=0.001, "Sense Resistance (Ohm)"=1.0} ("Transient"), "Sense Resistance (Ohm)"=w735, "Delay - t1 (s)"=w736, "Duration of the pulse (s)"=w737, "Delay - t2 (s)"=w738, "Load Current 1 - Iload1 (A)"=w739, "Load Current 2 - Iload2 (A)"=w740, "Slew rate A/us"=w741) -> (w742:T20)
            n303 = call "AWG Waveform Generator.vi"("FGEN Resource Name"=w744, "Transient"=w742, "Offset (V)"=w734, "error in (no error)"=w733) -> ("error out"=w745:errorcluster)  [unwired: 11 in]
          }
          frame True {
            # "Insufficient buffer and on-board memory"
          }
        }
      }
      frame "Test: Measure Transient" {
        n304 = Unbundle By Name(w770) -> ("Insufficient memory?"=w760:bool, "Scope Channels"=w758:string, "Test Inputs.Shunt Resistance (Ohm)"=w762:dbl, "Scope Acquired time(s)"=w757:dbl, "Test Pins.Measure Load Current"=w759:string)
        n305 = call "Progress Monitor.vi"("State"=w767) -> ("State Array Index"=w769:i32)  [unwired: 14 in]
        n306 = property on="Progress" class="Slide (strict)"(error in=w768, "Value"=w769) -> (error out=w761:errorcluster)  [unwired: 1 in, 1 out]
        n307 = case shown="False" w760 {
          tunnel: [w775 _] -> w766
          tunnel: [w786 _] -> w765
          tunnel: [w777 w789] -> w764
          tunnel: [w776 _] -> w763
          tunnel: w762 -> [w781 _]
          tunnel: w761 -> [w784 w789]
          tunnel: w758 -> [w782 _]
          tunnel: w759 -> [w780 _]
          tunnel: w757 -> [w779 _]
          frame False {
            # "5 multiples to have enough timeout"
            # "sufficient buffer and on-board memory and has valid sequence"
            n308 = call "Pin Name to Reference.vim"("Pin Name"=w780, "type"=refnum<k15> refnum ("instrument handle"), "error in (no error)"=w784) -> ("Reference"=w787:refnum<k15>, "error out"=w783:errorcluster)  [unwired: 7 in, 4 out]
            n309 = property class="niScope"(reference=w787, error in=w783) -> (reference out=w778:refnum<k15>, error out=w785:errorcluster, "Actual Sample Rate"=w786:dbl)
            n310 = Multiply(x=5.0, y=w779) -> (x*y=w773:dbl)
            n311 = call "Scope Measurement.vi"("Scope Reference"=w778, "Scope Channels"=w782, "Shunt Resistance"=w781, "error in (no error)"=w785, "Scope Timeout (s)"=w773) -> ("Measured Output Voltage"=w776:cluster{dbl[], dbl[]}, "Measured Load Current"=w775:cluster{dbl[], dbl[]}, "error out"=w777:errorcluster)  [unwired: 7 in, 1 out]
          }
          frame True {
            # "Insufficient buffer and on-board memory"
          }
        }
        n312 = Bundle By Name(cluster=w770, "Test Results.Measured Output Voltage"=w763, "Test Results.Measured Load Current"=w766, "Test Results.Actual Sample Rate in S/s"=w765) -> (w771:T17)
      }
      frame "Test: Calculate Out. Voltage Threshold" {
        # "Calculate reference Voltage Level for Settling time"
        n313 = call "Progress Monitor.vi"("State"=w790) -> ("State Array Index"=w793:i32)  [unwired: 14 in]
        n314 = property on="Progress" class="Slide (strict)"(error in=w791, "Value"=w793) -> (error out=w792:errorcluster)  [unwired: 1 in, 1 out]
        n315 = Unbundle By Name(w794) -> ("Test Inputs.Settling Time Calc Option"=w800:T11, "Test Inputs.Ref Voltage level for Settling Time Calc"=w799:dbl, "Test Inputs.% of Vnom for Settling Time Calc"=w798:dbl, "Test Inputs.Nominal Output Voltage in V"=w797:dbl)
        n316 = case shown="\"Percentage of Vnom\"" w800 {
          tunnel: w799 -> [w802 _]
          tunnel: w798 -> [_ w804]
          tunnel: w797 -> [_ w805]
          tunnel: [w802 w803] -> w796
          frame "Voltage Level ", Default {
          }
          frame "Percentage of Vnom" {
            n317 = formula code="y = (x/100)*v;"("x"=w804, "v"=w805) -> ("y"=w803:dbl)
          }
        }
        n318 = Bundle By Name(cluster=w794, "Test Inputs.Ref Voltage level for Settling Time Calc"=w796) -> (w795:T17)
      }
      frame "Test: Calculate Settling Time" {
        n319 = call "Progress Monitor.vi"("State"=w806) -> ("State Array Index"=w809:i32)  [unwired: 14 in]
        n320 = Unbundle By Name(w810) -> ("Output Voltage Coupling"=w812:i32, "Test Results.Measured Output Voltage.wfm"=w819:dbl[], "Test Inputs.Ref Voltage level for Settling Time Calc"=w818:dbl, "Test Inputs.Duration of the pulse in Second"=w817:dbl, "Test Results.Actual Sample Rate in S/s"=w816:dbl, "Test Inputs.Nominal Output Voltage in V"=w813:dbl)
        n321 = property on="Progress" class="Slide (strict)"(error in=w807, "Value"=w809) -> (error out=w808:errorcluster)  [unwired: 1 in, 1 out]
        n322 = call "CalculateSettlingTime.vi"("Waveform"=w819, "Waveform Coupling"=w812, "Recovery Volt Level (V)"=w818, "Duration of the pulse (s)"=w817, "Sampling Freq (S/s)"=w816, "DC Component (v)"=w813) -> ("FirstSpike. Duration (s)"=w815:dbl, "SecondSpike. Duration (s)"=w814:dbl)  [unwired: 8 in]
        n323 = Bundle By Name(cluster=w810, "Test Results.First Edge - Settling Time in s"=w815, "Test Results.Second Edge - Settling Time in s"=w814) -> (w811:T17)
      }
      frame "Test: Measure Slew Rate" {
        # "A/s to A/us"
        # "V to I conversion"
        n324 = Unbundle By Name(w838) -> ("Test Inputs.Shunt Resistance (Ohm)"=w821:dbl, "Test Inputs.Measure Rising Edge Slew Rate?"=w822:bool, "Scope Acquired time(s)"=w842:dbl, "Test Pins.Measure Load Current"=w845:string, "Test Inputs.Measure Falling Edge Slew Rate?"=w827:bool)
        n325 = call "Pin Name to Reference.vim"("Pin Name"=w845, "type"=refnum<k15> refnum ("instrument handle"), "error in (no error)"=w846) -> ("Reference"=w831:refnum<k15>, "Channel"=w843:string, "error out"=w828:errorcluster)  [unwired: 7 in, 3 out]
        n326 = Multiply(x=5.0, y=w842) -> (x*y=w840:dbl)
        n327 = case shown="True" w827 {
          tunnel: [w851 w853] -> w844
          tunnel: w843 -> [_ w860]
          tunnel: w840 -> [_ w859]
          tunnel: [nan w855] -> w836
          tunnel: w831 -> [_ w858]
          tunnel: w828 -> [w851 w857]
          tunnel: [FALSE ("Edge not found?") w852] -> w825
          frame False {
          }
          frame True {
            w861 = T27 1011 items=["None"=4000, "Frequency"=2, "Average Frequency"=1016, "FFT Frequency"=1008, "Period"=3, "Average Period"=1015, "Rise Time"=0, "Fall Time"=1, "Rising Slew Rate"=1010, "Falling Slew Rate"=1011, "Overshoot"=18, "Preshoot"=19, "Voltage RMS"=4, "Voltage Cycle RMS"=16, "AC Estimate"=1012, "FFT Amplitude"=1009, "Voltage Average"=10, "Voltage Cycle Average"=17, "DC Estimate"=1013, "Voltage Max"=6, "Voltage Min"=7, "Voltage Peak-to-Peak"=5, "Voltage High"=8, "Voltage Low"=9, "Voltage Amplitude"=15, "Voltage Top"=1007, "Voltage Base"=1006, "Voltage Base-to-Top"=1017, "Negative Width"=11, "Positive Width"=12, "Negative Duty Cycle"=13, "Positive Duty Cycle"=14, "Integral"=1005, "Area"=1003, "Cycle Area"=1004, "Time Delay"=1014, "Phase Delay"=1018, "Low Ref Volts"=1000, "Mid Ref Volts"=1001, "High Ref Volts"=1002, "Volt. Hist. Mean"=2000, "Volt. Hist. Stdev"=2001, "Volt. Hist. Median"=2003, "Volt. Hist. Mode"=2010, "Volt. Hist. Max"=2005, "Volt. Hist. Min"=2006, "Volt. Hist. Peak-to-Peak"=2002, "Volt. Hist. Mean + Stdev"=2007, "Volt. Hist. Mean + 2 Stdev"=2008, "Volt. Hist. Mean + 3 Stdev"=2009, "Volt. Hist. Hits"=2004, "Volt. Hist. New Hits"=2011, "Time Hist. Mean"=3000, "Time Hist. Stdev"=3001, "Time Hist. Median"=3003, "Time Hist. Mode"=3010, "Time Hist. Max"=3005, "Time Hist. Min"=3006, "Time Hist. Peak-to-Peak"=3002, "Time Hist. Mean + Stdev"=3007, "Time Hist. Mean + 2 Stdev"=3008, "Time Hist. Mean + 3 Stdev"=3009, "Time Hist. Hits"=3004, "Time Hist. New Hits"=3011] ("scalar measurement")
            n328 = call-poly <instrlib>:"niScope Fetch Measurement (poly).vi"("instrument handle"=w858, "timeout"=w859, "channels"=w860, "scalar measurement"=w861, "error in"=w857) -> ("result"=w856:dbl, "error out"=w854:errorcluster)  [unwired: 8 in, 1 out]
            n329 = call "SlewRate Validity.vi"("Measured Slew Rate"=w856, "error in (no error)"=w854) -> ("Slew rate Out"=w855:dbl, "Edge not found?"=w852:bool, "error out"=w853:errorcluster)  [unwired: 11 in]
          }
        }
        n330 = case shown="True" w822 {
          tunnel: w843 -> [_ w873]
          tunnel: w840 -> [_ w872]
          tunnel: [nan w867] -> w837
          tunnel: w831 -> [_ w871]
          tunnel: [w864 w868] -> w829
          tunnel: w828 -> [w864 w870]
          tunnel: [FALSE ("Edge not found?") w865] -> w826
          frame False {
          }
          frame True {
            w874 = T27 1010 items=["None"=4000, "Frequency"=2, "Average Frequency"=1016, "FFT Frequency"=1008, "Period"=3, "Average Period"=1015, "Rise Time"=0, "Fall Time"=1, "Rising Slew Rate"=1010, "Falling Slew Rate"=1011, "Overshoot"=18, "Preshoot"=19, "Voltage RMS"=4, "Voltage Cycle RMS"=16, "AC Estimate"=1012, "FFT Amplitude"=1009, "Voltage Average"=10, "Voltage Cycle Average"=17, "DC Estimate"=1013, "Voltage Max"=6, "Voltage Min"=7, "Voltage Peak-to-Peak"=5, "Voltage High"=8, "Voltage Low"=9, "Voltage Amplitude"=15, "Voltage Top"=1007, "Voltage Base"=1006, "Voltage Base-to-Top"=1017, "Negative Width"=11, "Positive Width"=12, "Negative Duty Cycle"=13, "Positive Duty Cycle"=14, "Integral"=1005, "Area"=1003, "Cycle Area"=1004, "Time Delay"=1014, "Phase Delay"=1018, "Low Ref Volts"=1000, "Mid Ref Volts"=1001, "High Ref Volts"=1002, "Volt. Hist. Mean"=2000, "Volt. Hist. Stdev"=2001, "Volt. Hist. Median"=2003, "Volt. Hist. Mode"=2010, "Volt. Hist. Max"=2005, "Volt. Hist. Min"=2006, "Volt. Hist. Peak-to-Peak"=2002, "Volt. Hist. Mean + Stdev"=2007, "Volt. Hist. Mean + 2 Stdev"=2008, "Volt. Hist. Mean + 3 Stdev"=2009, "Volt. Hist. Hits"=2004, "Volt. Hist. New Hits"=2011, "Time Hist. Mean"=3000, "Time Hist. Stdev"=3001, "Time Hist. Median"=3003, "Time Hist. Mode"=3010, "Time Hist. Max"=3005, "Time Hist. Min"=3006, "Time Hist. Peak-to-Peak"=3002, "Time Hist. Mean + Stdev"=3007, "Time Hist. Mean + 2 Stdev"=3008, "Time Hist. Mean + 3 Stdev"=3009, "Time Hist. Hits"=3004, "Time Hist. New Hits"=3011] ("scalar measurement")
            n331 = call-poly <instrlib>:"niScope Fetch Measurement (poly).vi"("instrument handle"=w871, "timeout"=w872, "channels"=w873, "scalar measurement"=w874, "error in"=w870) -> ("result"=w866:dbl, "error out"=w869:errorcluster)  [unwired: 8 in, 1 out]
            n332 = call "SlewRate Validity.vi"("Measured Slew Rate"=w866, "error in (no error)"=w869) -> ("Slew rate Out"=w867:dbl, "Edge not found?"=w865:bool, "error out"=w868:errorcluster)  [unwired: 11 in]
          }
        }
        n333 = Divide(x=w837, y=w821) -> (x/y=w824:dbl)
        n334 = Divide(x=w836, y=w821) -> (x/y=w823:dbl)
        n335 = Divide(x=w824, y=1000000.0) -> (x/y=w835:dbl)
        n336 = Divide(x=w823, y=1000000.0) -> (x/y=w833:dbl)
        n337 = Bundle By Name(cluster=w838, "Test Results.Rising Edge - Measured Slew Rate (A/us)"=w835, "Rising Edge not found?"=w826, "Test Results.Falling Edge - Measured Slew Rate (A/us)"=w833, "Falling Edge not found?"=w825) -> (w839:T17)
        n338 = Merge Errors(w829, w844) -> (w830:errorcluster)
      }
      frame "Test: Cleanup DCPower" {
        # "Cleanup Load SMU if valid"
        n339 = call "Progress Monitor.vi"("State"=w889) -> ("State Array Index"=w892:i32)  [unwired: 14 in]
        n340 = property on="Progress" class="Slide (strict)"(error in=w890, "Value"=w892) -> (error out=w891:errorcluster)  [unwired: 1 in, 1 out]
        n341 = Unbundle By Name(w895) -> ("Test Pins.Set Input Voltage"=w893:string, "Test Pins.Set Load Current"=w881:string)
        n342 = call "Pin Name to Reference.vim"("Pin Name"=w881, "type"=refnum<k15> refnum ("instrument handle"), "error in (no error)"=w891) -> ("Reference"=w879:refnum<k15>, "error out"=w878:errorcluster)  [unwired: 7 in, 4 out]
        n343 = call <instrlib>:"niDCPower Configure Output Enabled.vi"("error in (no error)"=w878, "output enabled"=FALSE, "instrument handle"=w879) -> ("error out"=w877:errorcluster, "instrument handle out"=w875:refnum<k15>)  [unwired: 7 in]
        n344 = call <instrlib>:"niDCPower Abort With Channels.vi"("error in (no error)"=w877, "instrument handle"=w875) -> ("error out"=w882:errorcluster)  [unwired: 8 in, 1 out]
        n345 = call "Pin Name to Reference.vim"("Pin Name"=w893, "type"=refnum<k15> refnum ("instrument handle"), "error in (no error)"=w882) -> ("Reference"=w886:refnum<k15>, "error out"=w887:errorcluster)  [unwired: 7 in, 4 out]
        n346 = call <instrlib>:"niDCPower Configure Output Enabled.vi"("error in (no error)"=w887, "output enabled"=FALSE, "instrument handle"=w886) -> ("error out"=w885:errorcluster, "instrument handle out"=w884:refnum<k15>)  [unwired: 7 in]
        n347 = call <instrlib>:"niDCPower Abort With Channels.vi"("error in (no error)"=w885, "instrument handle"=w884) -> ("error out"=w883:errorcluster)  [unwired: 8 in, 1 out]
      }
      frame "Test: Cleanup Scope" {
        w901 = FALSE
        n348 = call "Progress Monitor.vi"("State"=w906) -> ("State Array Index"=w909:i32)  [unwired: 14 in]
        n349 = property on="Progress" class="Slide (strict)"(error in=w907, "Value"=w909) -> (error out=w908:errorcluster)  [unwired: 1 in, 1 out]
        n350 = Unbundle By Name(w912) -> ("Test Pins.Measure Load Current"=w902:string, "Test Pins.Measure Output Voltage"=w911:string)
        n351 = call "Pin Name to Reference.vim"("Pin Name"=w911, "type"=refnum<k15> refnum ("instrument handle"), "error in (no error)"=w908) -> ("Reference"=w914:refnum<k15>, "Channel"=w913:string, "error out"=w915:errorcluster)  [unwired: 7 in, 3 out]
        n352 = property class="niScope"(reference=w914, error in=w915, "Active Channel"=w913, "Channel Enabled"=w901) -> (error out=w903:errorcluster)  [unwired: 1 out]
        n353 = call "Pin Name to Reference.vim"("Pin Name"=w902, "type"=refnum<k15> refnum ("instrument handle"), "error in (no error)"=w903) -> ("Reference"=w898:refnum<k15>, "Channel"=w897:string, "error out"=w899:errorcluster)  [unwired: 7 in, 3 out]
        n354 = property class="niScope"(reference=w898, error in=w899, "Active Channel"=w897, "Channel Enabled"=w901) -> (reference out=w905:refnum<k15>, error out=w904:errorcluster)
        n355 = call <instrlib>:"niScope Abort.vi"("instrument handle"=w905, "error in"=w904) -> ("error out"=w910:errorcluster)  [unwired: 12 in, 1 out]
      }
      frame "Test: Cleanup Fgen" {
        # "Disable Output and Abort"
        n356 = call "Progress Monitor.vi"("State"=w924) -> ("State Array Index"=w927:i32)  [unwired: 14 in]
        n357 = property on="Progress" class="Slide (strict)"(error in=w925, "Value"=w927) -> (error out=w926:errorcluster)  [unwired: 1 in, 1 out]
        n358 = Unbundle By Name(w929) -> ("Test Pins.Set Arbitrary Waveform"=w928:string)
        n359 = call "Pin Name to Reference.vim"("Pin Name"=w928, "type"=refnum<k15> refnum ("instrument handle"), "error in (no error)"=w926) -> ("Reference"=w922:refnum<k15>, "Channel"=w921:string, "error out"=w930:errorcluster)  [unwired: 7 in, 3 out]
        n360 = call <instrlib>:"niFgen Output Enable.vi"("error in (no error)"=w930, "Output Enable (default: True)"=FALSE, "Channel Name"=w921, "Instrument Handle"=w922) -> ("error out"=w923:errorcluster, "Instrument Handle Out"=w918:refnum<k15>)  [unwired: 6 in]
        n361 = call <instrlib>:"niFgen Abort Generation.vi"("error in (no error)"=w923, "Instrument Handle"=w918) -> ("error out"=w919:errorcluster)  [unwired: 8 in, 1 out]
      }
      frame "Test: Update UI" {
        # "If you want to update more indicators in the front panel do it here. It is efficient to update the UI in one case rather than in several cases. Also, it is a good practice to store the results in the data cluster in an efficient format and then get the data from data cluster and update the UI, in that way we could have the front panel independent of how we manipulate the data."
        n362 = call "Progress Monitor.vi"("State"=w940) -> ("State Array Index"=w943:i32)  [unwired: 14 in]
        n363 = Unbundle By Name(w947) -> ("Test Results.Measured Output Voltage"=w939:cluster{"x-axis":dbl[], "wfm":dbl[]}, "Test Results.Measured Load Current"=w937:cluster{"x-axis":dbl[], "wfm":dbl[]}, "Test Results"=→"Test Results":T15, "Test Results.First Edge - Settling Time in s"=→"First Edge - Settling Time (s)":dbl, "Test Results.Second Edge - Settling Time in s"=→"Second Edge - Settling Time (s)":dbl, "Test Results.Rising Edge - Measured Slew Rate (A/us)"=→"Rising Edge - Measured Slew Rate (A/us)":dbl, "Test Results.Falling Edge - Measured Slew Rate (A/us)"=→"Falling Edge - Measured Slew Rate (A/us)":dbl, "Falling Edge not found?"=→"Falling Edge not found?":bool, "Rising Edge not found?"=→"Rising Edge not found?":bool)
        n364 = property on="Progress" class="Slide (strict)"(error in=w941, "Value"=w943) -> (error out=w942:errorcluster)  [unwired: 1 in, 1 out]
        n365 = Build Array(w939, w937) -> (→"Load Transient":cluster{"x-axis":dbl[], "wfm":dbl[]}[])
      }
      frame "Test: End" {
        # "End of the Test Procedure. Do cleanup of resources or references."
        n366 = call "Progress Monitor.vi"("State"=w949) -> ("State Array Index"=w952:i32)  [unwired: 14 in]
        n367 = property on="Progress" class="Slide (strict)"(error in=w950, "Value"=w952) -> (error out=w951:errorcluster)  [unwired: 1 in, 1 out]
      }
      frame "---------------------Misc-----------------------" {
      }
      frame "Error" {
        # "Handle the error and make sure to clear the error."
        n368 = Unbundle By Name(w961) -> ("Termination Monitor Info.Caller Information.Mode"=w960:T8)
        n369 = case shown="\"MeasurementSuite\"" w960 {
          tunnel: w964 -> [w968 w973 w975]
          tunnel: [w966 w970 w974] -> w962
          tunnel: [_ TRUE _] -> w959
          tunnel: w958 -> [_ w971 _]
          frame "Standalone" {
            w965 = T28 2 items=["no dialog", "OK message", "continue or stop message", "OK message + warnings", "continue/stop + warnings"] ("type of dialog (OK msg:1)")
            n370 = call <vilib>:"General Error Handler.vi"("type of dialog (OK msg:1)"=w965, "error in (no error)"=w968) -> ("error out"=w967:errorcluster)  [unwired: 9 in, 4 out]
            n371 = call <vilib>:"Clear Errors.vi"("error in (no error)"=w967) -> ("error out"=w966:errorcluster)  [unwired: 5 in, 1 out]
          }
          frame "Automation" {
            n372 = call <userlib>:"Release.vi"("Queue in"=w971) -> ("Error Out"=w969:errorcluster)  [unwired: 14 in]
            n373 = Merge Errors(w973, w969) -> (w970:errorcluster)
          }
          frame "MeasurementSuite" {
            n374 = property on="ErrorOccured" class="Clust (strict)"("Val(Sgnl)"=w975) -> (error out=w974:errorcluster)  [unwired: 2 in, 1 out]
          }
        }
      }
      frame "Exit" {
        # "Last case called before stopping the execution. \nError occured in this state will not be captured by Error state."
        n375 = call <userlib>:"Release.vi"("Queue in"=w981, "Error In"=w982) -> ("Error Out"=w977:errorcluster)  [unwired: 13 in]
        n376 = property on="Progress" class="Slide (strict)"(error in=w977, "Visible"=FALSE) -> (error out=w976:errorcluster)  [unwired: 1 in, 1 out]
      }
    }
  }
  "error out" <- w4
  "Header" <- "Load Transient_AWG" ("Header")
